vi "信号发生器（配置文件1）.vi"() -> ()   [LabVIEW 2020]
uses:
  <vilib>/Utility/xml.llb/Read From XML File(string).vi
  <vilib>/Utility/config.llb/Read Key (I32).vi
  <vilib>/Utility/config.llb/Read Key (Double).vi
  <vilib>/Utility/config.llb/Read Key (Boolean).vi
  <vilib>/Utility/xml.llb/Write to XML File(string).vi
  <vilib>/Utility/config.llb/Write Key (U32).vi
  <vilib>/Utility/config.llb/Write Key (Double).vi
  <vilib>/Utility/config.llb/Write Key (Boolean).vi
  <vilib>/measure/NI_MABase.lvlib
  <vilib>/Utility/config.llb/NI_LVConfig.lvlib
panel:
  out "Hall Channel 1":waveform(dbl)(graph)
  out "车型数组":string[](array[string])
  in  "STOP":bool
  in  "AO3 Channel":u32(ring)=4 items=["Hall Channel 1", "Hall Channel 2", "ME Channel 1", "ME Channel 2", "ME Channel 3", "ME Channel 4"]
  in  "AO2 Channel":u32(ring)=3 items=["ME Channel 1", "ME Channel 2", "ME Channel 1", "ME Channel 2", "ME Channel 3", "ME Channel 4"]
  in  "AO1 Channel":u32(ring)=2 items=["Hall Channel 1", "Hall Channel 2", "ME Channel 1", "ME Channel 2", "ME Channel 3", "ME Channel 4"]
  in  "AO0 Channel":u32(ring) items=["Hall Channel 1", "Hall Channel 2", "ME Channel 1", "ME Channel 2", "ME Channel 3", "ME Channel 4"]
  out "转速表":dbl(knob) scale=0.0..3000.0
  in  "Speed FM":dbl(knob)=583.5936811226446 caption="转速调频" scale=50.0..1000.0
  in  "Brand":u32(ring)=2 items=["卡特", "凯斯", "日立", "神钢", "沃尔沃", "现代", "小松", "住友", "三一"]
  in  "Vehicle models":u32(ring) items=["五十铃6HK1", "五十铃6WG1", "五十铃新版4HK1"]
  out "ME Channel 4":waveform(dbl)(graph)
  out "ME Channel 3":dynamicdata(graph)
  out "ME Channel 2":waveform(dbl)(graph)
  out "ME Channel 1":dynamicdata(graph)
  out "Hall Channel 2":waveform(dbl)(graph)
  out "数组大小":i32
  out "品牌":string
  out "品牌数组":string[](array[string])
  in  "error":errorcluster caption="错误输入（无错误）"
  in  "字符串数组类型":string[](array[string])
  out "数值合法":bool
  out "凸轮轴参数":T1
  out "0凸轮轴信号类型":u32
  out "0凸轮轴电压幅值":dbl format="%#.1f"
  out "0信号个数":dbl=7.0 caption="信号个数" format="%#.1f"
  out "0凸轮轴个数":dbl=1.0 caption="凸轮轴个数" format="%#.1f"
  out "0凸轮轴是否取反":bool
  out "0凸轮轴周期":dbl=3.0 caption="凸轮轴周期" format="%#.1f"
  out "0起始偏移":dbl=3.0 caption="凸轮轴周期" format="%#.1f"
  out "0插齿间隔":dbl=3.0 caption="凸轮轴周期" format="%#.1f"
  out "0间隔齿数":dbl=3.0 caption="凸轮轴周期" format="%#.1f"
  out "曲轴参数":T2
  out "0曲轴轴信号类型":u32
  out "0曲轴电压幅值":dbl format="%#.1f"
  out "0总齿数":dbl=7.0 caption="信号个数" format="%#.1f"
  out "0曲轴个数":dbl=1.0 caption="凸轮轴个数" format="%#.1f"
  out "0曲轴是否取反":bool
  out "0缺齿数":dbl=3.0 caption="凸轮轴周期" format="%#.1f"
  out "0曲轴圈数":dbl=3.0 caption="凸轮轴周期" format="%#.1f"
  out "0缺齿偏移":dbl=3.0 caption="凸轮轴周期" format="%#.1f"
  out "品牌车型数组":string[](array[string])
  out "凸轮轴信号类型":u16(ring) items=["磁电式", "霍尔式", "无曲轴"]
  out "曲轴圈数信号":dynamicdata(graph)
  out "1缺齿偏移":dbl=4.0
  out "缺齿偏移":dbl=8.2 format="%_2f"
  out "长平组信号正弦":dynamicdata(graph)
  out "间隔长平+正弦信号":dynamicdata(graph)
  out "曲轴组合波形":waveform(dbl)(graph)
  out "1曲轴圈数":dbl=4.0
  out "曲轴圈数":dbl=8.2
  out "长平组信号":dynamicdata(graph)
  out "间隔长平+凸信号":dynamicdata(graph)
  out "间隔齿数":dbl=3.0
  out "1间隔齿数":dbl=3.0 caption="凸轮轴周期"
  out "1插齿间隔":dbl=3.0 caption="凸轮轴周期"
  out "1起始偏移":dbl=3.0 caption="凸轮轴周期"
  out "插齿间隔":dbl=8.2
  out "起始偏移":dbl=8.2
  out "车型数组大小":i32
  in  "error":errorcluster caption="错误输入（无错误）"
  in  "字符串数组类型":string[](array[string])
  out "凸轮轴周期·":dbl=8.2 caption="凸轮轴周期"
  out "凸轮轴个数":dbl=8.2
  out "曲轴个数":dbl=8.2
  out "信号个数":dbl=8.2
  out "凸轮轴是否取反":bool
  out "凸轮轴电压幅值":dbl=8.2 format="%0.2p"
  out "曲轴是否取反":bool
  out "曲轴信号类型":u16(ring) items=["磁电式", "霍尔式", "无曲轴"]
  out "缺齿数":dbl=4.0
  out "总齿数":dbl=60.0
  out "曲轴电压幅值":dbl=8.2 format="%0.2p"
  out "1凸轮轴周期·":dbl=3.0 caption="凸轮轴周期"
  out "1凸轮轴是否取反":bool
  out "1凸轮轴个数":dbl=1.0 caption="凸轮轴个数"
  out "1信号个数":dbl=7.0 caption="信号个数"
  out "1凸轮轴电压幅值":dbl=5.0 caption="凸轮轴电压幅值" format="%0.2p"
  out "1凸轮轴信号类型":u16(ring)=1 items=["磁电式", "霍尔式", "无凸轮轴"]
  out "1缺齿数":dbl=4.0
  out "1总齿数":dbl=60.0
  out "1曲轴个数":dbl=2.0 caption="曲轴个数"
  out "1曲轴是否取反":bool
  out "1曲轴电压幅值":dbl=18.0 caption="曲轴电压幅值" format="%0.2p"
  out "1曲轴信号类型":u16(ring) items=["磁电式", "霍尔式", "无曲轴"]
  out "1波形图":waveform(dbl)(graph)
  out "起始偏移（方波）":dbl
  out "起始偏移（正弦）":dbl=0.5
  out "中短平+2正弦":dynamicdata(graph)
  out "长平+1正弦":dynamicdata(graph)
  out "长水平线数量（正弦）":dbl
  out "一个正弦波形图":waveform(dbl)(graph)
  out "起始水平线个数（正弦）":dbl
  out "起始平+1正弦":dynamicdata(graph)
  out "6波形图":waveform(dbl)(graph)
  out "5波形图":waveform(dbl)(graph)
  out "起始水平线个数（方波）":dbl
  out "长平+1凸":dynamicdata(graph)
  out "长水平线数量（方波）":dbl
  out "曲轴":dynamicdata(graph)
  out "曲轴方波缺齿波形图":dynamicdata(graph)
  out "曲轴方波偏移量":dbl=8.2 format="%0.2p"
  out "曲轴方波波形图":waveform(dbl)(graph)
  out "中、短平+2凸":dynamicdata(graph)
  out "起始平+1凸":dynamicdata(graph)
  out "一个凸起波形图":dynamicdata(graph)
  out "曲轴正弦偏移量":dbl caption="偏移量" format="%0.2p"
  out "曲轴正弦波形图":waveform(dbl)(graph)
  out "完\n整\n缺\n齿\n波":waveform(dbl)(graph)
  out "未\n翻\n转\n半\n缺\n齿":dynamicdata(graph)
  out "圆\n弧\n+\n水\n平":dynamicdata(graph)
  out "半\n缺\n齿\n水\n平\n线":waveform(dbl)(graph)
  out "圆\n弧":waveform(dbl)(graph)
  out "t0":timestamp
  out "x轴取点间隔":dbl
  out "循环次数":i32
  out "圆弧点数":dbl=33.0 format="%0.2p"
  out "dt":dbl
  out "圆半径":dbl=2.48 format="%0.2p"
  out "部分\n正弦\n波形图":waveform(dbl)(graph)
  in  "波形发生率Fs":dbl=50000.0
types:
  T1 = cluster{"0凸轮轴信号类型":u32, "0凸轮轴电压幅值":dbl, "0信号个数":dbl, "0凸轮轴个数":dbl, "0凸轮轴是否取反":bool, "0凸轮轴周期":dbl, "0起始偏移":dbl, "0插齿间隔":dbl, "0间隔齿数":dbl}
  T2 = cluster{"0曲轴轴信号类型":u32, "0曲轴电压幅值":dbl, "0总齿数":dbl, "0曲轴个数":dbl, "0曲轴是否取反":bool, "0却齿数":dbl, "0曲轴圈数":dbl, "0缺齿偏移":dbl}
  T3 = typedef "NI_LVConfig.lvlib/Config Data RefNum.ctl" = refnum<k1>
  T4 = cluster{"0曲轴轴信号类型":u32, "0曲轴电压幅值":dbl, "0总齿数":dbl, "0曲轴个数":dbl, "0曲轴是否取反":bool, "0缺齿数":dbl, "0曲轴圈数":dbl, "0缺齿偏移":dbl}
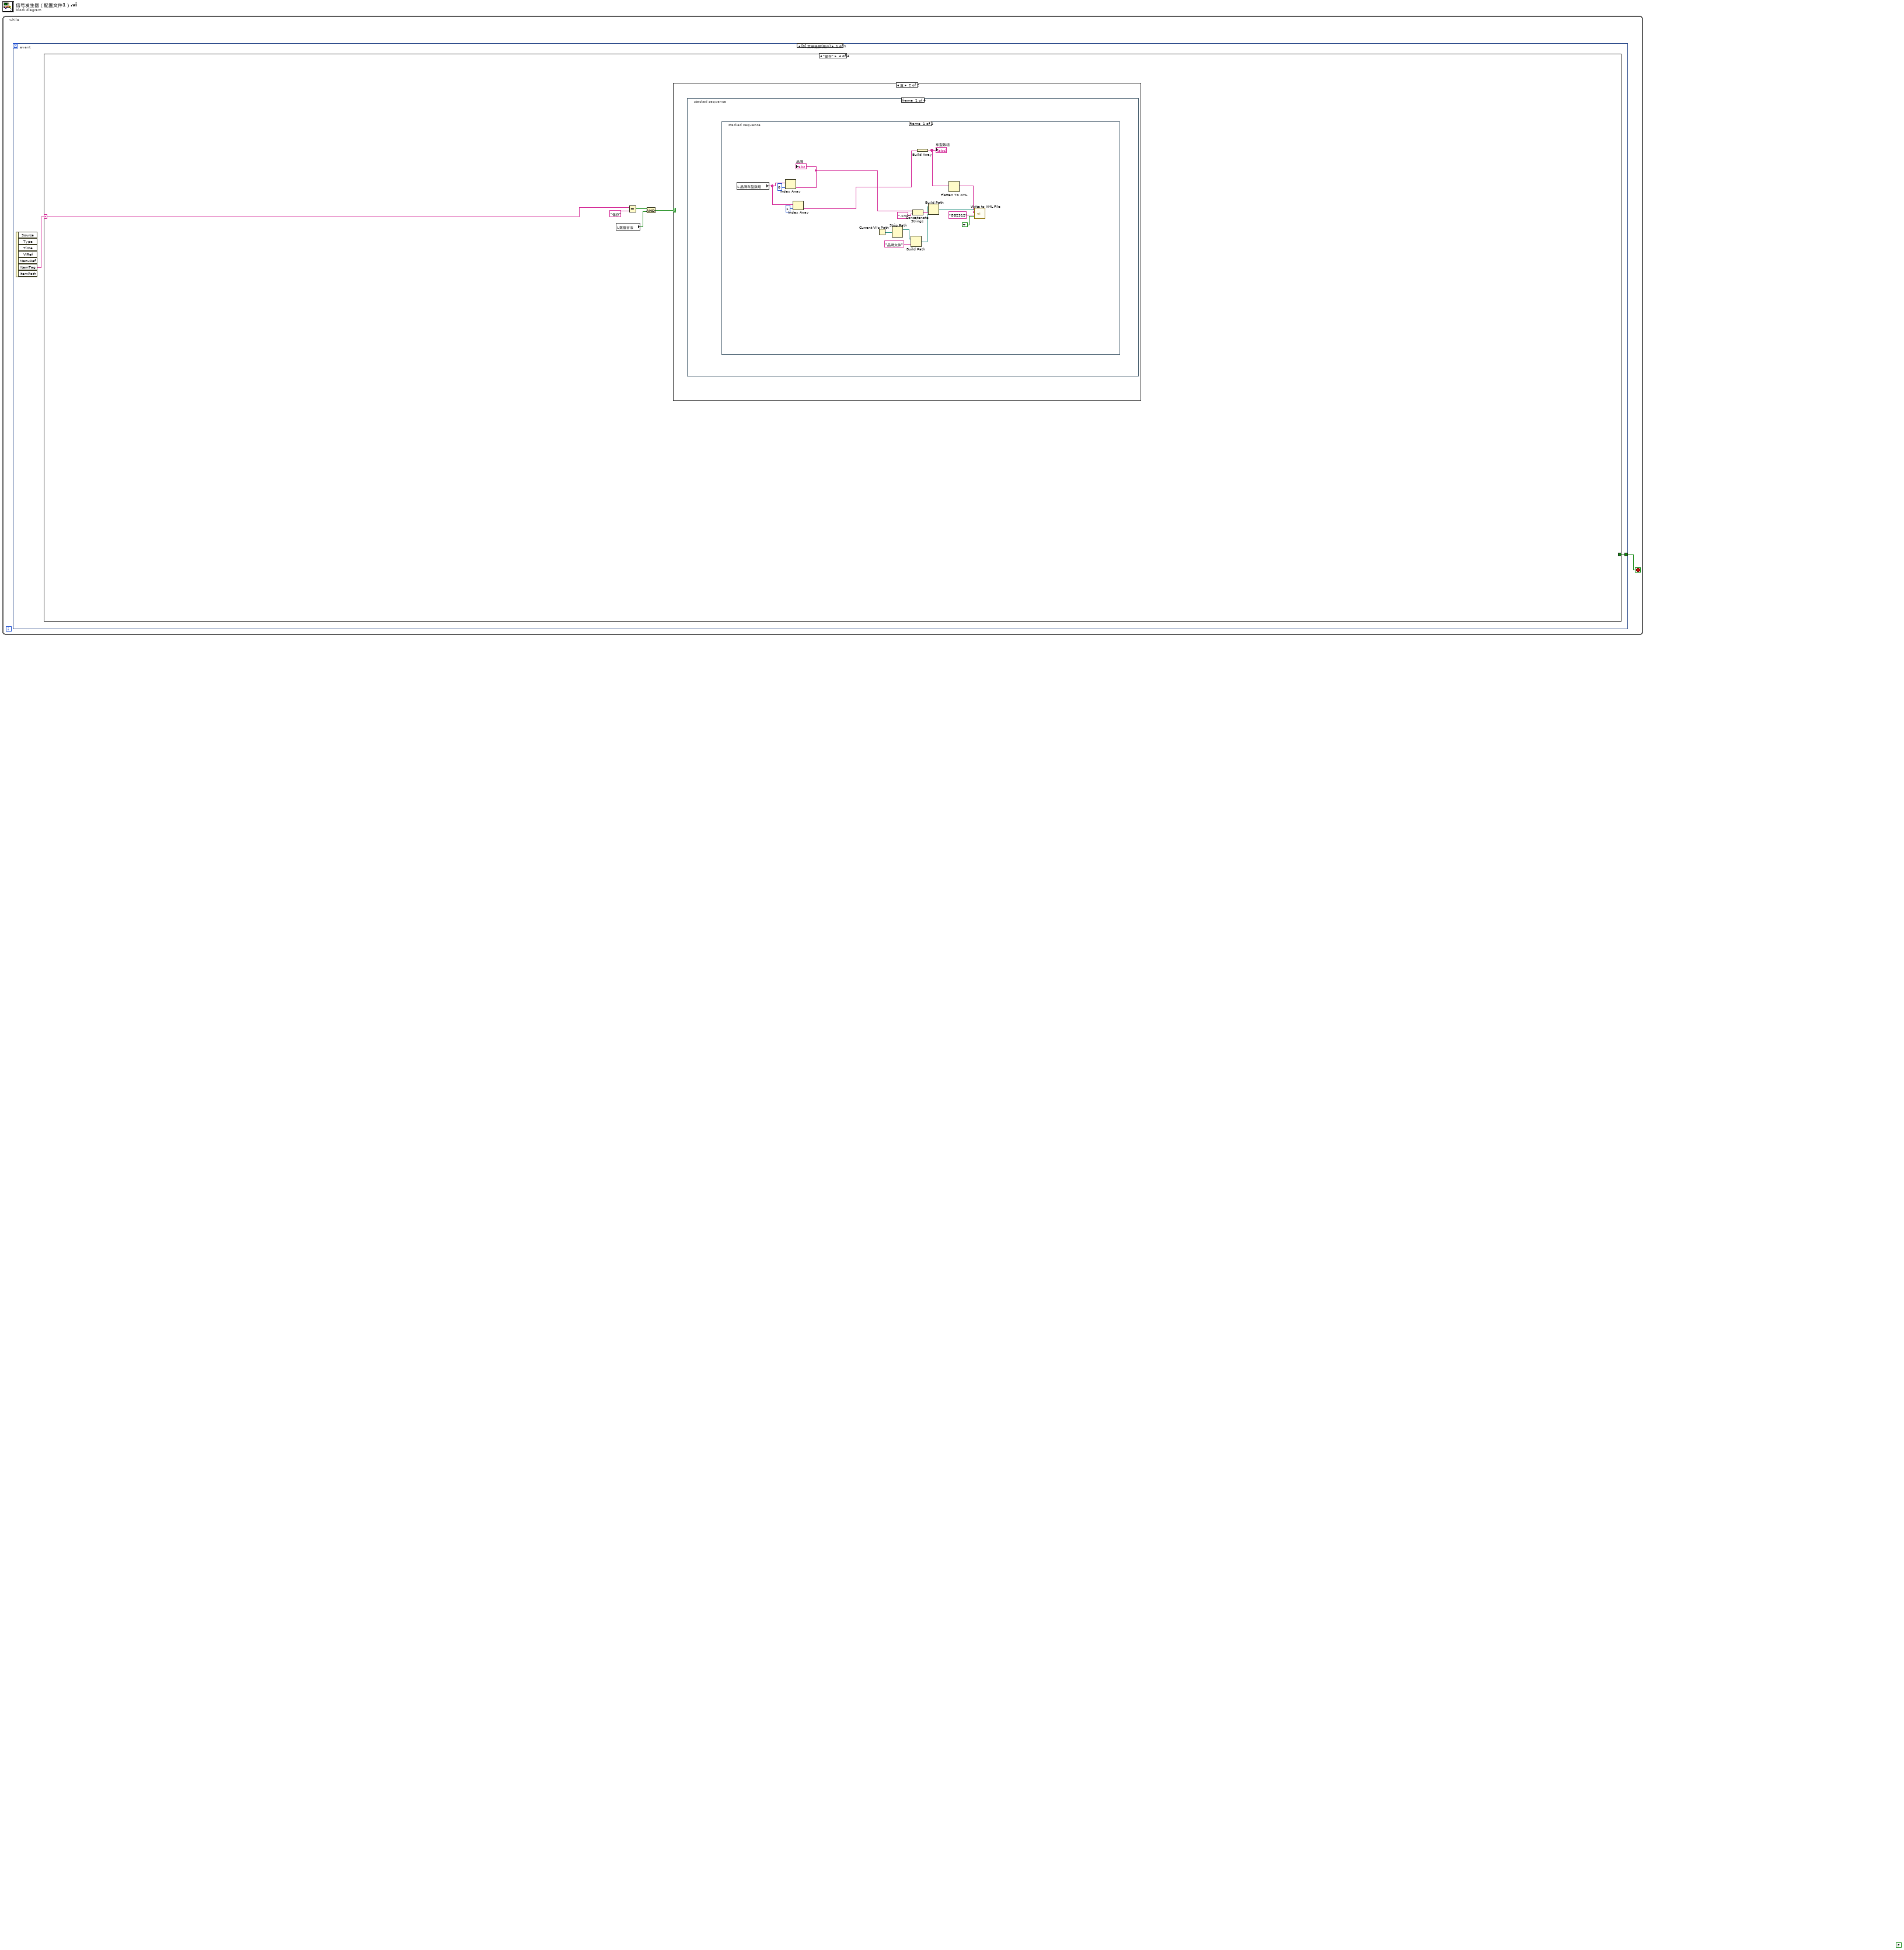
[diagram p0: block diagram]
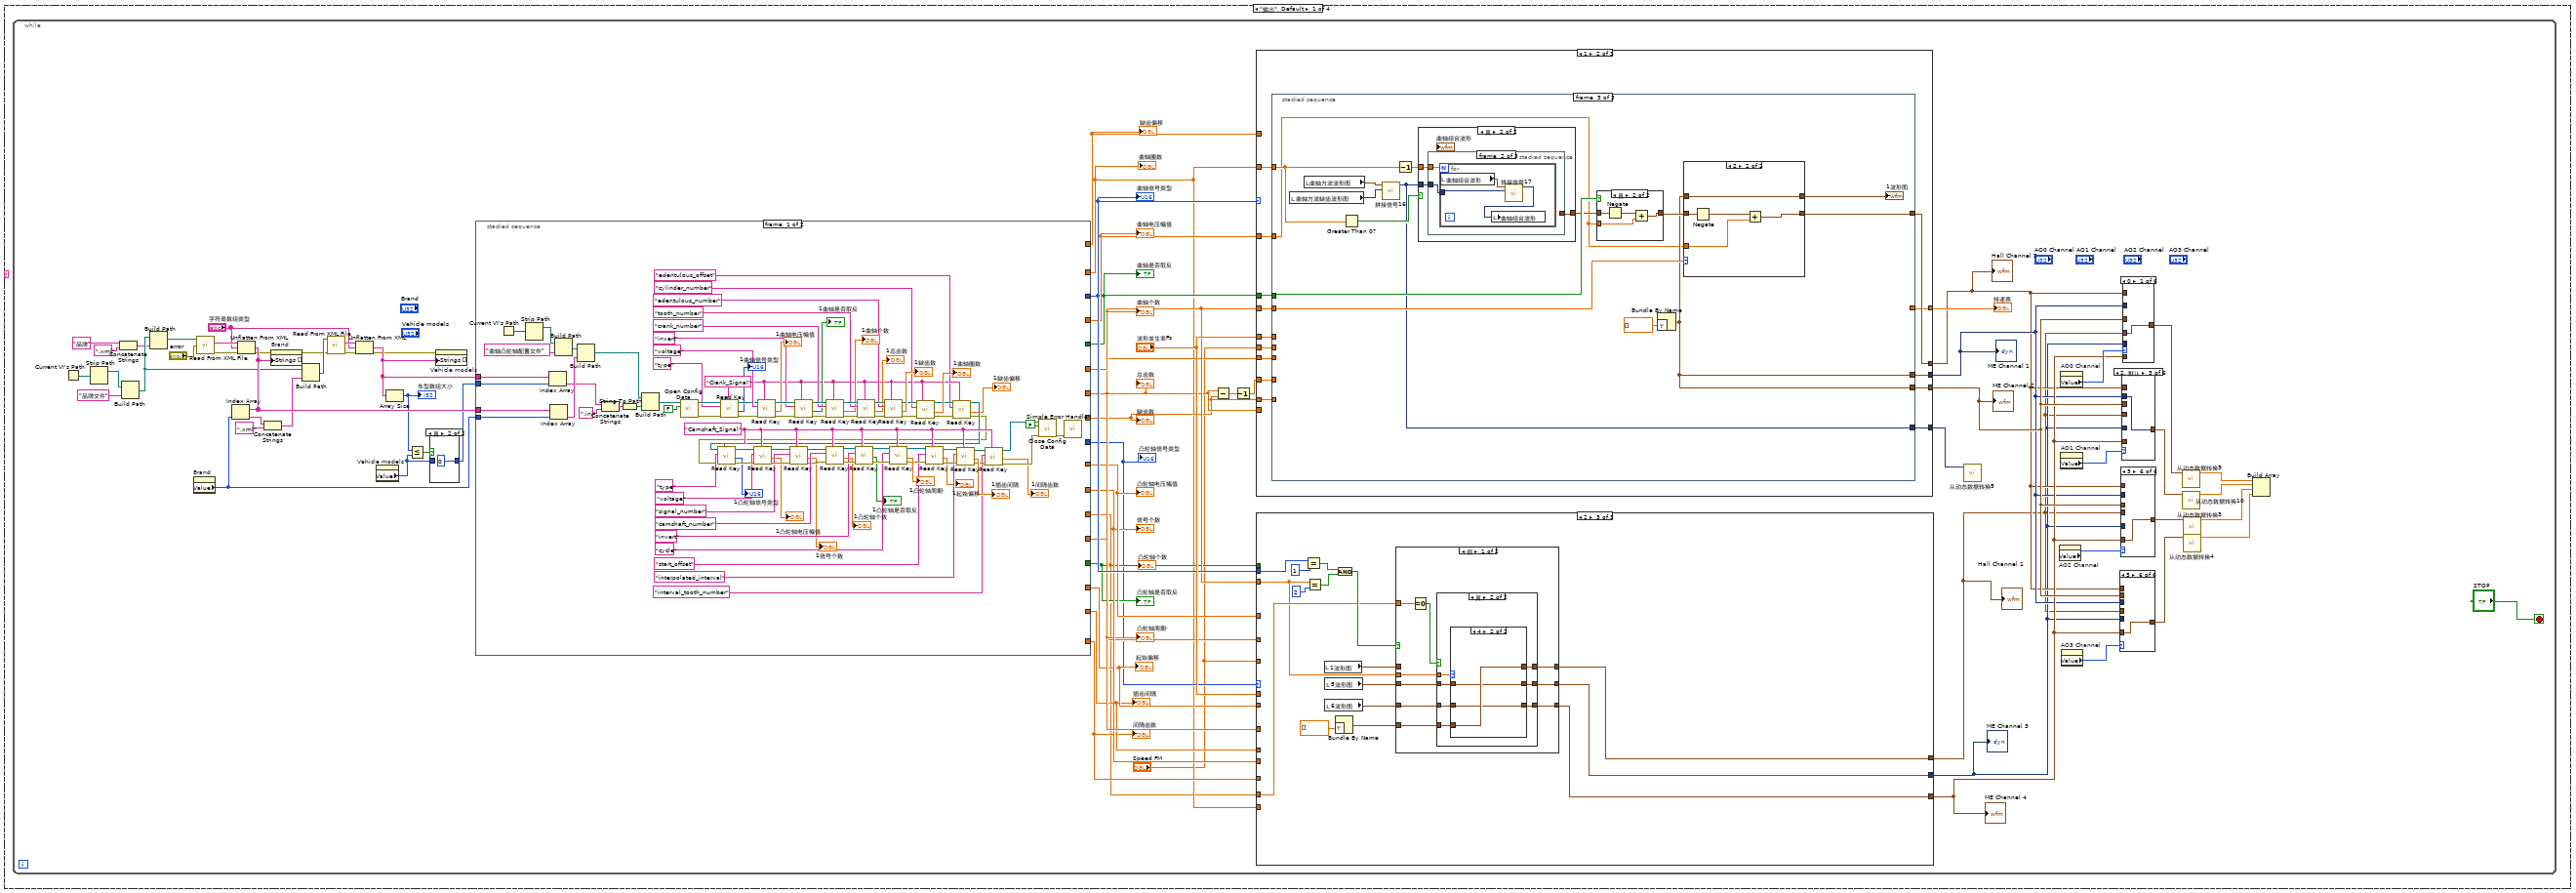
[diagram p2: hidden frame]
diagram:
  (unwired) FALSE
  n1 = while {
    stop <- w1 stop-if-true
    n2 = event shown="[0] 菜单选择(用户)" {
      selector: _ -> [_]
      dyn-events: _ -> [_]
      timeout: _ -> [_]
      tunnel: [w3] -> w1
      event Menu Selection (User) {
        n3 = event-data() -> ("ItemTag"=w2:string)  [unwired: 1 in, 6 out]
        n4 = case shown="\"保存\"" w2 {
          selector: w2 -> [_ _ _ w1190]
          tunnel: [_ TRUE _ _] -> w3
          frame "输出", Default {
            n5 = while {
              stop <- "STOP" stop-if-true
              n6 = Current VI's Path() -> (path=w53:path)
              n7 = Strip Path(path=w53) -> (stripped path=w52:path)  [unwired: 1 out]
              n8 = Concatenate Strings("品牌" ("字符串"), ".xml") -> (w43:string)
              n9 = Build Path(base path=w52, name or relative path="品牌文件" ("名称或相对路径")) -> (appended path=w44:path)
              n10 = Build Path(base path=w44, name or relative path=w43) -> (appended path=w42:path)
              n11 = property on="Brand" class="Ring (严格)"() -> ("Value"=w59:u32)  [unwired: 2 in, 2 out]
              n12 = call-poly <vilib>:"Read From XML File.vi"("error in (no error)"="error", "XML File Path"=w42) -> ("error out"=w56:errorcluster, "XML Elements"=w55:string)  [unwired: 7 in, 1 out]
              n13 = Unflatten From XML(xml string=w55, type="字符串数组类型", error in (no error)=w56) -> (value=w60:string[], error out=w48:errorcluster)
              n14 = Index Array(array=w60, index=w59) -> (element=w54:string)
              n15 = Concatenate Strings(w54, ".xml") -> (w51:string)
              n16 = property on="Brand" class="Ring (严格)"(error in=w48, "Strings []"=w60) -> (error out=w13:errorcluster)  [unwired: 1 in, 1 out]
              n17 = Build Path(base path=w44, name or relative path=w51) -> (appended path=w37:path)
              n18 = call-poly <vilib>:"Read From XML File.vi"("error in (no error)"=w13, "XML File Path"=w37) -> ("error out"=w41:errorcluster, "XML Elements"=w40:string)  [unwired: 7 in, 1 out]
              n19 = Unflatten From XML(xml string=w40, type="字符串数组类型", error in (no error)=w41) -> (value=w58:string[], error out=w39:errorcluster)
              n20 = property on="Vehicle models" class="Ring (严格)"() -> ("Value"=w35:u32)  [unwired: 2 in, 2 out]
              n21 = Array Size(array=w58) -> (size(s)=w34:i32)
              "车型数组大小" <- w34
              n22 = Less Or Equal?(x=w34, y=w35) -> (x <= y?=w36:bool)
              n23 = case shown="真" w36 {
                tunnel: w35 -> [w98 _]
                tunnel: [w98 0] -> w57
                frame False {
                }
                frame True {
                }
              }
              n24 = property on="Vehicle models" class="Ring (严格)"(error in=w39, "Strings []"=w58) -> ()  [unwired: 1 in, 2 out]
              n25 = stacked-sequence {
                tunnel: [_ w206] -> w70
                tunnel: [_ w205] -> w69
                tunnel: [_ w204] -> w68
                tunnel: [_ w203] -> w67
                tunnel: [_ w202] -> w66
                tunnel: [_ w201] -> w65
                tunnel: [_ w200] -> w22
                tunnel: [_ w199] -> w64
                tunnel: [_ w198] -> w63
                tunnel: [_ w197] -> w10
                tunnel: [_ w196] -> w62
                tunnel: [_ w195] -> w61
                tunnel: w60 -> [w134 _]
                tunnel: w58 -> [w131 _]
                tunnel: w59 -> [w127 _]
                tunnel: w57 -> [w126 _]
                tunnel: [_ w194] -> w33
                tunnel: [_ w193] -> w32
                tunnel: [_ w192] -> w31
                tunnel: [_ w191] -> w11
                tunnel: [_ w190] -> w30
                frame #0 {
                  w113 = "Camshaft_Signal" ("section")
                  w103 = "Crank_Signal" ("section")
                  n26 = Current VI's Path() -> (path=w140:path)
                  n27 = Strip Path(path=w140) -> (stripped path=w139:path)  [unwired: 1 out]
                  n28 = Index Array(array=w131, index=w126) -> (element=w130:string)
                  n29 = Index Array(array=w134, index=w127) -> (element=w133:string)
                  n30 = Build Path(base path=w139, name or relative path="曲轴凸轮轴配置文件" ("名称或相对路径")) -> (appended path=w135:path)
                  n31 = Build Path(base path=w135, name or relative path=w133) -> (appended path=w136:path)
                  n32 = Concatenate Strings(w130, ".ini" ("字符串")) -> (w128:string)
                  n33 = String To Path(string=w128) -> (path=w129:path)
                  n34 = Build Path(base path=w136, name or relative path=w129) -> (appended path=w137:path)
                  n35 = call <vilib>:"Open Config Data.vi"("create file if necessary (T)"=FALSE ("create file if necessary? (T)"), "configuration file path"=w137) -> ("error out"=w169:errorcluster, "refnum"=w167:T3)  [unwired: 7 in, 1 out]
                  n36 = call-poly <vilib>:"Read Key.vi"("section"=w103, "error in (no error)"=w169, "key"="type", "refnum"=w167) -> ("error out"=w170:errorcluster, "value"=→"1曲轴信号类型":i32, "refnum out"=w168:T3)  [unwired: 1 in, 4 out]
                  n37 = call-poly <vilib>:"Read Key.vi"("section"=w103, "error in (no error)"=w170, "key"="voltage" ("键2"), "refnum"=w168) -> ("error out"=w165:errorcluster, "value"=→"1曲轴电压幅值":dbl, "refnum out"=w164:T3)  [unwired: 1 in, 4 out]
                  n38 = call-poly <vilib>:"Read Key.vi"("section"=w103, "error in (no error)"=w165, "key"="invert" ("键3"), "refnum"=w164) -> ("error out"=w162:errorcluster, "value"=→"1曲轴是否取反":bool, "refnum out"=w161:T3)  [unwired: 1 in, 4 out]
                  n39 = call-poly <vilib>:"Read Key.vi"("section"=w103, "error in (no error)"=w162, "key"="crank_number" ("键3"), "refnum"=w161) -> ("error out"=w159:errorcluster, "value"=→"1曲轴个数":dbl, "refnum out"=w158:T3)  [unwired: 1 in, 4 out]
                  n40 = call-poly <vilib>:"Read Key.vi"("section"=w103, "error in (no error)"=w159, "key"="tooth_number" ("键3"), "refnum"=w158) -> ("error out"=w156:errorcluster, "value"=→"1总齿数":dbl, "refnum out"=w157:T3)  [unwired: 1 in, 4 out]
                  n41 = call-poly <vilib>:"Read Key.vi"("section"=w103, "error in (no error)"=w156, "key"="edentulous_number" ("键3"), "refnum"=w157) -> ("error out"=w109:errorcluster, "value"=→"1缺齿数":dbl, "refnum out"=w108:T3)  [unwired: 1 in, 4 out]
                  n42 = call-poly <vilib>:"Read Key.vi"("section"=w103, "error in (no error)"=w109, "key"="cylinder_number" ("键3"), "refnum"=w108) -> ("error out"=w102:errorcluster, "value"=→"1曲轴圈数":dbl, "refnum out"=w105:T3)  [unwired: 1 in, 4 out]
                  n43 = call-poly <vilib>:"Read Key.vi"("section"=w103, "error in (no error)"=w102, "key"="edentulous_offset" ("键2"), "refnum"=w105) -> ("error out"=w101:errorcluster, "value"=→"1缺齿偏移":dbl, "refnum out"=w106:T3)  [unwired: 1 in, 4 out]
                  n44 = call-poly <vilib>:"Read Key.vi"("section"=w113, "error in (no error)"=w101, "key"="type" ("键3"), "refnum"=w106) -> ("error out"=w189:errorcluster, "value"=→"1凸轮轴信号类型":i32, "refnum out"=w188:T3)  [unwired: 2 in, 3 out]
                  n45 = call-poly <vilib>:"Read Key.vi"("section"=w113, "error in (no error)"=w189, "key"="voltage" ("键3"), "refnum"=w188) -> ("error out"=w182:errorcluster, "value"=→"1凸轮轴电压幅值":dbl, "refnum out"=w180:T3)  [unwired: 2 in, 3 out]
                  n46 = call-poly <vilib>:"Read Key.vi"("section"=w113, "error in (no error)"=w182, "key"="signal_number" ("键3"), "refnum"=w180) -> ("error out"=w145:errorcluster, "value"=→"1信号个数":dbl, "refnum out"=w179:T3)  [unwired: 2 in, 3 out]
                  n47 = call-poly <vilib>:"Read Key.vi"("section"=w113, "error in (no error)"=w145, "key"="camshaft_number" ("键3"), "refnum"=w179) -> ("error out"=w181:errorcluster, "value"=→"1凸轮轴个数":dbl, "refnum out"=w178:T3)  [unwired: 2 in, 3 out]
                  n48 = call-poly <vilib>:"Read Key.vi"("section"=w113, "error in (no error)"=w181, "key"="invert" ("键2"), "refnum"=w178) -> ("error out"=w183:errorcluster, "value"=→"1凸轮轴是否取反":bool, "refnum out"=w177:T3)  [unwired: 2 in, 3 out]
                  n49 = call-poly <vilib>:"Read Key.vi"("section"=w113, "error in (no error)"=w183, "key"="cycle", "refnum"=w177) -> ("error out"=w122:errorcluster, "value"=→"1凸轮轴周期·":dbl, "refnum out"=w125:T3)  [unwired: 2 in, 3 out]
                  n50 = call-poly <vilib>:"Read Key.vi"("section"=w113, "error in (no error)"=w122, "key"="start_offset" ("键2"), "refnum"=w125) -> ("error out"=w123:errorcluster, "value"=→"1起始偏移":dbl, "refnum out"=w124:T3)  [unwired: 2 in, 3 out]
                  n51 = call-poly <vilib>:"Read Key.vi"("section"=w113, "error in (no error)"=w123, "key"="interpolated_interval", "refnum"=w124) -> ("error out"=w116:errorcluster, "value"=→"1插齿间隔":dbl, "refnum out"=w117:T3)  [unwired: 2 in, 3 out]
                  n52 = call-poly <vilib>:"Read Key.vi"("section"=w113, "error in (no error)"=w116, "key"="interval_tooth_number", "refnum"=w117) -> ("error out"=w115:errorcluster, "value"=→"1间隔齿数":dbl, "refnum out"=w114:T3)  [unwired: 2 in, 3 out]
                  n53 = call <vilib>:"Close Config Data.vi"("error in (no error)"=w115, "write file if changed (T)"=FALSE ("write configuration file? (T)"), "refnum"=w114) -> ("error out"=w184:errorcluster)  [unwired: 8 out]
                  n54 = call <vilib>:"Simple Error Handler.vi"("error in (no error)"=w184) -> ()  [unwired: 1 in, 8 out]
                }
                frame #1 {
                  n55 = local read "1缺齿偏移"() -> (w190:dbl)
                  n56 = local read "1曲轴圈数"() -> (w191:dbl)
                  n57 = local read "1曲轴信号类型"() -> (w206:u16)
                  n58 = local read "1曲轴电压幅值"() -> (w205:dbl)
                  n59 = local read "1曲轴是否取反"() -> (w204:bool)
                  n60 = local read "1曲轴个数"() -> (w203:dbl)
                  n61 = local read "1总齿数"() -> (w202:dbl)
                  n62 = local read "1缺齿数"() -> (w201:dbl)
                  n63 = local read "1凸轮轴信号类型"() -> (w200:u16)
                  n64 = local read "1凸轮轴电压幅值"() -> (w199:dbl)
                  n65 = local read "1信号个数"() -> (w198:dbl)
                  n66 = local read "1凸轮轴个数"() -> (w197:dbl)
                  n67 = local read "1凸轮轴周期·"() -> (w195:dbl)
                  n68 = local read "1凸轮轴是否取反"() -> (w196:bool)
                  n69 = local read "1起始偏移"() -> (w194:dbl)
                  n70 = local read "1插齿间隔"() -> (w193:dbl)
                  n71 = local read "1间隔齿数"() -> (w192:dbl)
                }
              }
              "总齿数" <- w66
              "缺齿数" <- w65
              "曲轴信号类型" <- w70
              "曲轴电压幅值" <- w69
              "曲轴是否取反" <- w68
              "凸轮轴电压幅值" <- w64
              "凸轮轴是否取反" <- w62
              "信号个数" <- w63
              "曲轴个数" <- w67
              "凸轮轴个数" <- w10
              "凸轮轴周期·" <- w61
              "起始偏移" <- w33
              "插齿间隔" <- w32
              "间隔齿数" <- w31
              "曲轴圈数" <- w11
              "缺齿偏移" <- w30
              "凸轮轴信号类型" <- w22
              n72 = Subtract(x=w66, y=w65) -> (x-y=w73:dbl)
              n73 = Decrement(x=w73) -> (x-1=w72:dbl)
              n74 = case shown="2" w22 {
                tunnel: "Speed FM" -> [w220 w398 _]
                tunnel: "波形发生率Fs" -> [w219 w397 _]
                tunnel: w66 -> [w218 w396 _]
                tunnel: w64 -> [w221 w395 _]
                tunnel: [w212 w394 w644] -> w4
                tunnel: w63 -> [w217 w393 _]
                tunnel: [w213 w392 w641] -> w20
                tunnel: [w214 w391 w640] -> w6
                tunnel: w61 -> [w216 w387 _]
                tunnel: w10 -> [w215 w390 w639]
                tunnel: w70 -> [_ _ w651]
                tunnel: w67 -> [_ _ w636]
                tunnel: w62 -> [w211 w389 _]
                tunnel: w33 -> [w210 w384 _]
                tunnel: w32 -> [w209 w385 _]
                tunnel: w31 -> [w207 w383 _]
                tunnel: w11 -> [w208 _ _]
                frame 0, Default {
                  n75 = stacked-sequence {
                    tunnel: w221 -> [w249 _ _ w327]
                    tunnel: w220 -> [w231 w260 w284 w339]
                    tunnel: w219 -> [w238 w259 w283 w340]
                    tunnel: w218 -> [w246 _ _ _]
                    tunnel: w217 -> [w247 _ _ w312]
                    tunnel: w216 -> [w229 _ w276 _]
                    tunnel: w215 -> [_ _ _ w331]
                    tunnel: [_ _ _ w330] -> w214
                    tunnel: [_ _ _ w328] -> w213
                    tunnel: [_ _ _ w325] -> w212
                    tunnel: w211 -> [_ _ _ w321]
                    tunnel: w210 -> [w224 w255 _ _]
                    tunnel: w209 -> [_ _ w273 _]
                    tunnel: w208 -> [w222 _ _ _]
                    tunnel: w207 -> [_ _ _ w311]
                    frame #0 {
                      n76 = Divide(x=w231, y=w229) -> (x/y=w230:dbl)
                      n77 = Decrement(x=w247) -> (x-1=w223:dbl)
                      n78 = Divide(x=w249, y=2.0) -> (x/y=w237:dbl)
                      n79 = Divide(x=w238, y=w230) -> (x/y=w248:dbl)
                      n80 = Multiply(x=w246, y=w222) -> (x*y=w228:dbl)
                      n81 = Multiply(x=w229, y=w223) -> (x*y=w227:dbl)
                      n82 = Subtract(x=w228, y=w227) -> (x-y=w226:dbl)
                      n83 = Bundle By Name(cluster=cluster{"Fs":dbl, "#s":dbl} {"Fs"=1000.0, "#s"=1000.0} ("sampling info"), "Fs"=w238, "#s"=w248) -> (w253:cluster{"Fs":dbl, "#s":dbl})
                      n84 = Divide(x=w226, y=w223) -> (x/y=w225:dbl)
                      n85 = Subtract(x=w225, y=w224) -> (x-y=w239:dbl)
                      "起始水平线个数（正弦）" <- w239
                      n86 = call <vilib>:"Sine Waveform.vi"("offset"=0.0, "sampling info"=w253, "reset signal"=TRUE, "amplitude"=w237, "frequency"=w230) -> ("signal out"=w232:waveform(dbl))  [unwired: 5 in, 1 out]
                      "一个正弦波形图" <- w232
                      n87 = Divide(x=w238, y=w231) -> (x/y=w243:dbl)
                      n88 = Multiply(x=w243, y=w239) -> (x*y=w242:dbl)
                      n89 = Bundle By Name(cluster=cluster{"Fs":dbl, "#s":dbl} {"Fs"=1000.0, "#s"=1000.0} ("sampling info"), "Fs"=w238, "#s"=w242) -> (w244:cluster{"Fs":dbl, "#s":dbl})
                      n90 = call <vilib>:"Square Waveform.vi"("duty cycle (%)"=0.0, "offset"=0.0, "sampling info"=w244, "reset signal"=TRUE, "amplitude"=0.0, "frequency"=w231) -> ("signal out"=w235:waveform(dbl))  [unwired: 4 in, 1 out]
                      n91 = call "拼接信号25"("Input Signal B"=w232, "Input Signal A"=w235) -> ("Appended Signals"=→"起始平+1正弦":dynamicdata)  [unwired: 8 in, 1 out]
                      "起始偏移（正弦）" <- w224
                    }
                    frame #1 {
                      n92 = local read "起始水平线个数（正弦）"() -> (w270:dbl)
                      n93 = Divide(x=w259, y=w260) -> (x/y=w267:dbl)
                      n94 = Add(x=w270, y=w255) -> (x+y=w261:dbl)
                      "长水平线数量（正弦）" <- w261
                      n95 = Multiply(x=w267, y=w261) -> (x*y=w266:dbl)
                      n96 = Bundle By Name(cluster=cluster{"Fs":dbl, "#s":dbl} {"Fs"=1000.0, "#s"=1000.0} ("sampling info"), "Fs"=w259, "#s"=w266) -> (w268:cluster{"Fs":dbl, "#s":dbl})
                      n97 = call <vilib>:"Square Waveform.vi"("duty cycle (%)"=0.0, "offset"=0.0, "sampling info"=w268, "reset signal"=TRUE, "amplitude"=0.0, "frequency"=w260) -> ("signal out"=w258:waveform(dbl))  [unwired: 4 in, 1 out]
                      n98 = local read "一个正弦波形图"() -> (w257:waveform(dbl))
                      n99 = call "拼接信号26"("Input Signal B"=w257, "Input Signal A"=w258) -> ("Appended Signals"=→"长平+1正弦":dynamicdata)  [unwired: 8 in, 1 out]
                    }
                    frame #2 {
                      n100 = local read "长水平线数量（正弦）"() -> (w282:dbl)
                      n101 = local read "一个正弦波形图"() -> (w272:waveform(dbl))
                      n102 = Equal To 0?(x=w273) -> (x = 0?=w274:bool)
                      n103 = Subtract(x=w282, y=w276) -> (x-y=w275:dbl)
                      n104 = case shown="假" w274 {
                        tunnel: w284 -> [_ w299]
                        tunnel: w283 -> [_ w298]
                        tunnel: w273 -> [_ w297]
                        tunnel: w272 -> [w293 w296]
                        tunnel: [w293 w294] -> w271
                        frame True {
                        }
                        frame False {
                          n105 = Divide(x=w298, y=w299) -> (x/y=w305:dbl)
                          n106 = Multiply(x=w305, y=w297) -> (x*y=w304:dbl)
                          n107 = Bundle By Name(cluster=cluster{"Fs":dbl, "#s":dbl} {"Fs"=1000.0, "#s"=1000.0} ("sampling info"), "Fs"=w298, "#s"=w304) -> (w306:cluster{"Fs":dbl, "#s":dbl})
                          n108 = call <vilib>:"Square Waveform.vi"("duty cycle (%)"=0.0, "offset"=0.0, "sampling info"=w306, "reset signal"=TRUE, "amplitude"=0.0, "frequency"=w299) -> ("signal out"=w295:waveform(dbl))  [unwired: 4 in, 1 out]
                          n109 = call "拼接信号28"("Input Signal B"=w296, "Input Signal A"=w295) -> ("Appended Signals"=w294:dynamicdata)  [unwired: 8 in, 1 out]
                        }
                      }
                      n110 = Divide(x=w283, y=w284) -> (x/y=w290:dbl)
                      n111 = Subtract(x=w275, y=w273) -> (x-y=w281:dbl)
                      n112 = Multiply(x=w290, y=w281) -> (x*y=w289:dbl)
                      n113 = Bundle By Name(cluster=cluster{"Fs":dbl, "#s":dbl} {"Fs"=1000.0, "#s"=1000.0} ("sampling info"), "Fs"=w283, "#s"=w289) -> (w291:cluster{"Fs":dbl, "#s":dbl})
                      n114 = call <vilib>:"Square Waveform.vi"("duty cycle (%)"=0.0, "offset"=0.0, "sampling info"=w291, "reset signal"=TRUE, "amplitude"=0.0, "frequency"=w284) -> ("signal out"=w279:waveform(dbl))  [unwired: 4 in, 1 out]
                      n115 = local read "一个正弦波形图"() -> (w280:waveform(dbl))
                      n116 = call "拼接信号27"("Input Signal B"=w280, "Input Signal A"=w279) -> ("Appended Signals"=w278:dynamicdata)  [unwired: 8 in, 1 out]
                      n117 = call "拼接信号29"("Input Signal B"=w271, "Input Signal A"=w278) -> ("Appended Signals"=→"中短平+2正弦":dynamicdata)  [unwired: 8 in, 1 out]
                    }
                    frame #3 {
                      n118 = local read "起始偏移（正弦）"() -> (w332:dbl)
                      n119 = Greater Or Equal?(x=w311, y=2.0) -> (x >= y?=w308:bool)
                      n120 = case shown="真" w308 {
                        tunnel: [w358 w363] -> w310
                        tunnel: w311 -> [w357 w362]
                        frame False {
                          n121 = case shown="1, 默认" w357 {
                            tunnel: [w359] -> w358
                            frame 1, Default {
                              n122 = local read "中短平+2正弦"() -> (w360:dynamicdata)
                              n123 = local read "起始平+1正弦"() -> (w361:dynamicdata)
                              n124 = call "拼接信号19"("Input Signal B"=w360, "Input Signal A"=w361) -> ("Appended Signals"=w359:dynamicdata)  [unwired: 8 in, 1 out]
                            }
                          }
                        }
                        frame True {
                          n125 = stacked-sequence {
                            tunnel: [_ _ w372] -> w363
                            tunnel: w362 -> [_ w366 _]
                            frame #0 {
                              n126 = local read "起始平+1正弦"() -> (w364:dynamicdata)
                              n127 = local write "间隔长平+正弦信号"(w364) -> ()
                            }
                            frame #1 {
                              n128 = Decrement(x=w366) -> (x-1=w365:dbl)
                              n129 = for {
                                N: w365 -> [_]
                                n130 = local read "间隔长平+正弦信号"() -> (w369:dynamicdata)
                                n131 = local read "长平+1正弦"() -> (w368:dynamicdata)
                                n132 = call "拼接信号30"("Input Signal B"=w368, "Input Signal A"=w369) -> ("Appended Signals"=w367:dynamicdata)  [unwired: 8 in, 1 out]
                                n133 = local write "间隔长平+正弦信号"(w367) -> ()
                              }
                            }
                            frame #2 {
                              n134 = local read "间隔长平+正弦信号"() -> (w371:dynamicdata)
                              n135 = local read "中短平+2正弦"() -> (w370:dynamicdata)
                              n136 = call "拼接信号31"("Input Signal B"=w370, "Input Signal A"=w371) -> ("Appended Signals"=w372:dynamicdata)  [unwired: 8 in, 1 out]
                            }
                          }
                        }
                      }
                      n137 = Divide(x=w340, y=w339) -> (x/y=w346:dbl)
                      n138 = Multiply(x=w346, y=w332) -> (x*y=w345:dbl)
                      n139 = Bundle By Name(cluster=cluster{"Fs":dbl, "#s":dbl} {"Fs"=1000.0, "#s"=1000.0} ("sampling info"), "Fs"=w340, "#s"=w345) -> (w347:cluster{"Fs":dbl, "#s":dbl})
                      n140 = call <vilib>:"Square Waveform.vi"("duty cycle (%)"=0.0, "offset"=0.0, "sampling info"=w347, "reset signal"=TRUE, "amplitude"=0.0, "frequency"=w339) -> ("signal out"=w333:waveform(dbl))  [unwired: 4 in, 1 out]
                      n141 = local read "长平+1正弦"() -> (w334:dynamicdata)
                      n142 = Subtract(x=w312, y=4.0) -> (x-y=w318:dbl)
                      n143 = Decrement(x=w311) -> (x-1=w317:dbl)
                      n144 = Subtract(x=w318, y=w317) -> (x-y=w315:dbl)
                      n145 = Greater Or Equal?(x=w315, y=1.0) -> (x >= y?=w314:bool)
                      n146 = Decrement(x=w315) -> (x-1=w313:dbl)
                      n147 = call "拼接信号32"("Input Signal B"=w333, "Input Signal A"=w334) -> ("Appended Signals"=w338:dynamicdata)  [unwired: 8 in, 1 out]
                      n148 = case shown="真" w314 {
                        tunnel: w313 -> [_ w350]
                        tunnel: [_ w349] -> w309
                        frame False {
                        }
                        frame True {
                          n149 = stacked-sequence {
                            tunnel: w350 -> [_ w352 _]
                            tunnel: [_ _ w356] -> w349
                            frame #0 {
                              n150 = local read "长平+1正弦"() -> (w351:dynamicdata)
                              n151 = local write "长平组信号正弦"(w351) -> ()
                            }
                            frame #1 {
                              n152 = for {
                                N: w352 -> [_]
                                n153 = local read "长平组信号正弦"() -> (w355:dynamicdata)
                                n154 = local read "长平+1正弦"() -> (w354:dynamicdata)
                                n155 = call "拼接信号33"("Input Signal B"=w354, "Input Signal A"=w355) -> ("Appended Signals"=w353:dynamicdata)  [unwired: 8 in, 1 out]
                                n156 = local write "长平组信号正弦"(w353) -> ()
                              }
                            }
                            frame #2 {
                              n157 = local read "长平组信号正弦"() -> (w356:dynamicdata)
                            }
                          }
                        }
                      }
                      n158 = call "拼接信号34"("Input Signal B"=w309, "Input Signal A"=w310) -> ("Appended Signals"=w337:dynamicdata)  [unwired: 8 in, 1 out]
                      n159 = Bundle By Name("Y"=dbl[] []) -> (w326:waveform(dbl))  [unwired: 1 in]
                      n160 = call "拼接信号35"("Input Signal B"=w338, "Input Signal A"=w337) -> ("Appended Signals"=w324:dynamicdata)  [unwired: 8 in, 1 out]
                      n161 = case shown="真" w321 {
                        tunnel: [w373 w375] -> w323
                        tunnel: w324 -> [w373 w374]
                        frame False {
                        }
                        frame True {
                          n162 = Negate(x=w374) -> (-x=w375:dynamicdata)
                        }
                      }
                      n163 = Divide(x=w327, y=2.0) -> (x/y=w335:dbl)
                      n164 = Add(x=w335, y=w323) -> (x+y=w322:dynamicdata)
                      n165 = case shown="2, 默认" w331 {
                        tunnel: w322 -> [w377 w380]
                        tunnel: [w377 w380] -> w330
                        tunnel: [w376 w381] -> w328
                        tunnel: w327 -> [_ w379]
                        tunnel: w326 -> [w376 w378]
                        tunnel: [w376 w378] -> w325
                        frame 1 {
                        }
                        frame 2, Default {
                          n166 = Negate(x=w380) -> (-x=w382:dynamicdata)
                          n167 = Add(x=w382, y=w379) -> (x+y=w381:dynamicdata)
                        }
                      }
                    }
                  }
                }
                frame 1 {
                  n168 = Not Equal?(x=w387, y=1.0) -> (x != y?=w386:bool)
                  n169 = case shown="真" w386 {
                    tunnel: w398 -> [w407 w451]
                    tunnel: w397 -> [w419 w450]
                    tunnel: w396 -> [_ w449]
                    tunnel: w395 -> [w399 w448]
                    tunnel: [w417 w447] -> w394
                    tunnel: w393 -> [w420 w446]
                    tunnel: [w415 w445] -> w392
                    tunnel: [w415 w444] -> w391
                    tunnel: w390 -> [_ w443]
                    tunnel: w389 -> [w414 w442]
                    tunnel: w387 -> [w403 w441]
                    tunnel: w385 -> [_ w440]
                    tunnel: w384 -> [_ w439]
                    tunnel: w383 -> [_ w438]
                    frame False {
                      n170 = Divide(x=w399, y=2.0) -> (x/y=w400:dbl)
                      n171 = Divide(x=w419, y=w407) -> (x/y=w423:dbl)
                      n172 = Divide(x=w419, y=w407) -> (x/y=w404:dbl)
                      n173 = Multiply(x=w423, y=w420) -> (x*y=w422:dbl)
                      n174 = Bundle By Name(cluster=cluster{"Fs":dbl, "#s":dbl} {"Fs"=1000.0, "#s"=1000.0} ("sampling info"), "Fs"=w419, "#s"=w422) -> (w428:cluster{"Fs":dbl, "#s":dbl})
                      n175 = Multiply(x=w404, y=w403) -> (x*y=w405:dbl)
                      n176 = Bundle By Name(cluster=cluster{"Fs":dbl, "#s":dbl} {"Fs"=1000.0, "#s"=1000.0} ("sampling info"), "Fs"=w419, "#s"=w405) -> (w412:cluster{"Fs":dbl, "#s":dbl})
                      n177 = call <vilib>:"Square Waveform.vi"("duty cycle (%)"=50.0, "offset"=0.0, "sampling info"=w428, "reset signal"=TRUE, "amplitude"=w400, "frequency"=w407) -> ("signal out"=w421:waveform(dbl))  [unwired: 4 in, 1 out]
                      n178 = call <vilib>:"Square Waveform.vi"("duty cycle (%)"=0.0, "offset"=0.0, "sampling info"=w412, "reset signal"=TRUE, "amplitude"=0.0, "frequency"=w407) -> ("signal out"=w408:waveform(dbl))  [unwired: 4 in, 1 out]
                      n179 = case shown="真" w414 {
                        tunnel: w421 -> [w435 w437]
                        tunnel: [w435 w436] -> w402
                        frame False {
                        }
                        frame True {
                          n180 = Negate(x=w437) -> (-x=w436:waveform(dbl))
                        }
                      }
                      n181 = case shown="真" w414 {
                        tunnel: w408 -> [w430 w434]
                        tunnel: [w430 w433] -> w418
                        tunnel: w399 -> [_ w431]
                        frame False {
                        }
                        frame True {
                          n182 = Negate(x=w434) -> (-x=w432:waveform(dbl))
                          n183 = Add(x=w431, y=w432) -> (x+y=w433:waveform(dbl))
                        }
                      }
                      n184 = Add(x=w400, y=w402) -> (x+y=w401:waveform(dbl))
                      n185 = Bundle By Name("Y"=dbl[] []) -> (w415:waveform(dbl))  [unwired: 1 in]
                      n186 = call "拼接信号38"("Input Signal B"=w418, "Input Signal A"=w401) -> ("Appended Signals"=w417:dynamicdata)  [unwired: 8 in, 1 out]
                    }
                    frame True {
                      n187 = stacked-sequence {
                        tunnel: w451 -> [w456 w515 w525 w539 w597]
                        tunnel: w450 -> [w474 w514 w524 w540 w596]
                        tunnel: w449 -> [_ w517 _ _ _]
                        tunnel: w448 -> [w473 w516 w521 w549 w598]
                        tunnel: [_ _ _ _ w587] -> w447
                        tunnel: w446 -> [_ w513 _ _ w575]
                        tunnel: [_ _ _ _ w584] -> w445
                        tunnel: [_ _ _ _ w583] -> w444
                        tunnel: w441 -> [w453 w500 _ w538 _]
                        tunnel: w443 -> [_ _ _ _ w576]
                        tunnel: w442 -> [_ _ _ _ w579]
                        tunnel: w440 -> [_ _ _ w536 _]
                        tunnel: w439 -> [_ w493 w518 _ _]
                        tunnel: w438 -> [_ _ _ _ w572]
                        frame #0 {
                          n188 = Divide(x=w473, y=2.0) -> (x/y=w457:dbl)
                          n189 = Greater?(x=w453, y=2.0) -> (0:w452:bool)
                          n190 = Divide(x=w474, y=w456) -> (x/y=w455:dbl)
                          n191 = case shown="真" w452 {
                            tunnel: w474 -> [_ w488]
                            tunnel: [_ w484] -> w464
                            tunnel: w457 -> [_ w481]
                            tunnel: w456 -> [_ w480]
                            tunnel: w455 -> [_ w478]
                            tunnel: w453 -> [_ w475]
                            frame False {
                            }
                            frame True {
                              n192 = Subtract(x=w475, y=2.0) -> (x-y=w477:dbl)
                              n193 = Multiply(x=w478, y=w477) -> (x*y=w479:dbl)
                              n194 = Bundle By Name(cluster=cluster{"Fs":dbl, "#s":dbl} {"Fs"=1000.0, "#s"=1000.0} ("sampling info"), "Fs"=w488, "#s"=w479) -> (w486:cluster{"Fs":dbl, "#s":dbl})
                              n195 = call <vilib>:"Square Waveform.vi"("duty cycle (%)"=100.0, "offset"=0.0, "sampling info"=w486, "reset signal"=TRUE, "amplitude"=w481, "frequency"=w480) -> ("signal out"=w484:waveform(dbl))  [unwired: 4 in, 1 out]
                            }
                          }
                          n196 = Bundle By Name(cluster=cluster{"Fs":dbl, "#s":dbl} {"Fs"=1000.0, "#s"=1000.0} ("sampling info"), "Fs"=w474, "#s"=w455) -> (w471:cluster{"Fs":dbl, "#s":dbl})
                          n197 = call <vilib>:"Square Waveform.vi"("duty cycle (%)"=50.0, "offset"=0.0, "sampling info"=w471, "reset signal"=TRUE, "amplitude"=w457, "frequency"=w456) -> ("signal out"=w462:waveform(dbl))  [unwired: 4 in, 1 out]
                          n198 = call "从动态数据转换2"("Dynamic Data Type"=w462) -> ("Array"=w469:dbl[])  [unwired: 3 in]
                          n199 = Unbundle By Name(w462) -> ("t0"=w467:timestamp, "dt"=w468:dbl)  [unwired: 1 out]
                          n200 = Reverse 1D Array(array=w469) -> (reversed array=w470:dbl[])
                          n201 = Bundle By Name("Y"=w470, "t0"=w467, "dt"=w468) -> (w465:waveform(dbl))  [unwired: 1 in]
                          n202 = case shown="3, 默认" w453 {
                            tunnel: w465 -> [w491 w492]
                            tunnel: w464 -> [w490 _]
                            tunnel: [w489 w492] -> w463
                            frame 3, Default {
                              n203 = call "拼接信号5"("Input Signal B"=w490, "Input Signal A"=w491) -> ("Appended Signals"=w489:dynamicdata)  [unwired: 8 in, 1 out]
                            }
                            frame 2 {
                            }
                          }
                          n204 = call "拼接信号6"("Input Signal B"=w462, "Input Signal A"=w463) -> ("Appended Signals"=→"一个凸起波形图":dynamicdata)  [unwired: 8 in, 1 out]
                        }
                        frame #1 {
                          n205 = Decrement(x=w513) -> (x-1=w494:dbl)
                          n206 = Multiply(x=w517, y=2.0) -> (x*y=w499:dbl)
                          n207 = Multiply(x=w500, y=w494) -> (x*y=w498:dbl)
                          n208 = Subtract(x=w499, y=w498) -> (x-y=w496:dbl)
                          n209 = Divide(x=w516, y=2.0) -> (x/y=w502:dbl)
                          n210 = Divide(x=w514, y=w515) -> (x/y=w510:dbl)
                          n211 = Divide(x=w496, y=w494) -> (x/y=w495:dbl)
                          n212 = Subtract(x=w495, y=w493) -> (x-y=w504:dbl)
                          "起始水平线个数（方波）" <- w504
                          n213 = Multiply(x=w510, y=w504) -> (x*y=w509:dbl)
                          n214 = Bundle By Name(cluster=cluster{"Fs":dbl, "#s":dbl} {"Fs"=1000.0, "#s"=1000.0} ("sampling info"), "Fs"=w514, "#s"=w509) -> (w511:cluster{"Fs":dbl, "#s":dbl})
                          n215 = call <vilib>:"Square Waveform.vi"("duty cycle (%)"=0.0, "sampling info"=w511, "reset signal"=TRUE, "amplitude"=w502, "frequency"=w515) -> ("signal out"=w508:waveform(dbl))  [unwired: 5 in, 1 out]
                          n216 = local read "一个凸起波形图"() -> (w507:dynamicdata)
                          n217 = call "拼接信号8"("Input Signal B"=w507, "Input Signal A"=w508) -> ("Appended Signals"=→"起始平+1凸":dynamicdata)  [unwired: 8 in, 1 out]
                          "起始偏移（方波）" <- w493
                        }
                        frame #2 {
                          n218 = local read "起始水平线个数（方波）"() -> (w526:dbl)
                          n219 = Divide(x=w521, y=2.0) -> (x/y=w519:dbl)
                          n220 = Add(x=w518, y=w526) -> (x+y=w527:dbl)
                          "长水平线数量（方波）" <- w527
                          n221 = Divide(x=w524, y=w525) -> (x/y=w533:dbl)
                          n222 = Multiply(x=w533, y=w527) -> (x*y=w532:dbl)
                          n223 = Bundle By Name(cluster=cluster{"Fs":dbl, "#s":dbl} {"Fs"=1000.0, "#s"=1000.0} ("sampling info"), "Fs"=w524, "#s"=w532) -> (w534:cluster{"Fs":dbl, "#s":dbl})
                          n224 = local read "一个凸起波形图"() -> (w528:dynamicdata)
                          n225 = call <vilib>:"Square Waveform.vi"("duty cycle (%)"=0.0, "offset"=0.0, "sampling info"=w534, "reset signal"=TRUE, "amplitude"=w519, "frequency"=w525) -> ("signal out"=w529:waveform(dbl))  [unwired: 4 in, 1 out]
                          n226 = call "拼接信号22"("Input Signal B"=w528, "Input Signal A"=w529) -> ("Appended Signals"=→"长平+1凸":dynamicdata)  [unwired: 8 in, 1 out]
                        }
                        frame #3 {
                          n227 = local read "长水平线数量（方波）"() -> (w542:dbl)
                          n228 = Divide(x=w549, y=2.0) -> (x/y=w548:dbl)
                          n229 = Subtract(x=w542, y=w538) -> (x-y=w537:dbl)
                          n230 = Subtract(x=w537, y=w536) -> (x-y=w557:dbl)
                          n231 = Divide(x=w540, y=w539) -> (x/y=w541:dbl)
                          n232 = Multiply(x=w541, y=w557) -> (x*y=w562:dbl)
                          n233 = Multiply(x=w541, y=w536) -> (x*y=w553:dbl)
                          n234 = Bundle By Name(cluster=cluster{"Fs":dbl, "#s":dbl} {"Fs"=1000.0, "#s"=1000.0} ("sampling info"), "Fs"=w540, "#s"=w562) -> (w564:cluster{"Fs":dbl, "#s":dbl})
                          n235 = Bundle By Name(cluster=cluster{"Fs":dbl, "#s":dbl} {"Fs"=1000.0, "#s"=1000.0} ("sampling info"), "Fs"=w540, "#s"=w553) -> (w555:cluster{"Fs":dbl, "#s":dbl})
                          n236 = call <vilib>:"Square Waveform.vi"("duty cycle (%)"=0.0, "offset"=0.0, "sampling info"=w555, "reset signal"=TRUE, "amplitude"=w548, "frequency"=w539) -> ("signal out"=w543:waveform(dbl))  [unwired: 4 in, 1 out]
                          n237 = call <vilib>:"Square Waveform.vi"("duty cycle (%)"=0.0, "offset"=0.0, "sampling info"=w564, "reset signal"=TRUE, "amplitude"=w548, "frequency"=w539) -> ("signal out"=w561:waveform(dbl))  [unwired: 4 in, 1 out]
                          n238 = local read "一个凸起波形图"() -> (w560:dynamicdata)
                          n239 = local read "一个凸起波形图"() -> (w547:dynamicdata)
                          n240 = call "拼接信号11"("Input Signal B"=w560, "Input Signal A"=w561) -> ("Appended Signals"=w546:dynamicdata)  [unwired: 8 in, 1 out]
                          n241 = call "拼接信号12"("Input Signal B"=w547, "Input Signal A"=w543) -> ("Appended Signals"=w545:dynamicdata)  [unwired: 8 in, 1 out]
                          n242 = call "拼接信号10"("Input Signal B"=w545, "Input Signal A"=w546) -> ("Appended Signals"=→"中、短平+2凸":dynamicdata)  [unwired: 8 in, 1 out]
                        }
                        frame #4 {
                          n243 = local read "起始偏移（方波）"() -> (w582:dbl)
                          n244 = Divide(x=w598, y=2.0) -> (x/y=w594:dbl)
                          n245 = Divide(x=w596, y=w597) -> (x/y=w603:dbl)
                          n246 = Greater Or Equal?(x=w572, y=2.0) -> (x >= y?=w577:bool)
                          n247 = Multiply(x=w603, y=w582) -> (x*y=w602:dbl)
                          n248 = case shown="真" w577 {
                            tunnel: [w615 w620] -> w591
                            tunnel: w572 -> [w614 w619]
                            frame False {
                              n249 = case shown="1, 默认" w614 {
                                tunnel: [w616] -> w615
                                frame 1, Default {
                                n250 = local read "中、短平+2凸"() -> (w617:dynamicdata)
                                n251 = local read "起始平+1凸"() -> (w618:dynamicdata)
                                n252 = call "拼接信号4"("Input Signal B"=w617, "Input Signal A"=w618) -> ("Appended Signals"=w616:dynamicdata)  [unwired: 8 in, 1 out]
                                }
                              }
                            }
                            frame True {
                              n253 = stacked-sequence {
                                tunnel: [_ _ w629] -> w620
                                tunnel: w619 -> [_ w623 _]
                                frame #0 {
                                n254 = local read "起始平+1凸"() -> (w621:dynamicdata)
                                n255 = local write "间隔长平+凸信号"(w621) -> ()
                                }
                                frame #1 {
                                n256 = Decrement(x=w623) -> (x-1=w622:dbl)
                                n257 = for {
                                N: w622 -> [_]
                                n258 = local read "间隔长平+凸信号"() -> (w626:dynamicdata)
                                n259 = local read "长平+1凸"() -> (w625:dynamicdata)
                                n260 = call "拼接信号7"("Input Signal B"=w625, "Input Signal A"=w626) -> ("Appended Signals"=w624:dynamicdata)  [unwired: 8 in, 1 out]
                                n261 = local write "间隔长平+凸信号"(w624) -> ()
                                }
                                }
                                frame #2 {
                                n262 = local read "间隔长平+凸信号"() -> (w628:dynamicdata)
                                n263 = local read "中、短平+2凸"() -> (w627:dynamicdata)
                                n264 = call "拼接信号9"("Input Signal B"=w627, "Input Signal A"=w628) -> ("Appended Signals"=w629:dynamicdata)  [unwired: 8 in, 1 out]
                                }
                              }
                            }
                          }
                          n265 = Bundle By Name(cluster=cluster{"Fs":dbl, "#s":dbl} {"Fs"=1000.0, "#s"=1000.0} ("sampling info"), "Fs"=w596, "#s"=w602) -> (w604:cluster{"Fs":dbl, "#s":dbl})
                          n266 = call <vilib>:"Square Waveform.vi"("duty cycle (%)"=0.0, "offset"=0.0, "sampling info"=w604, "reset signal"=TRUE, "amplitude"=w594, "frequency"=w597) -> ("signal out"=w592:waveform(dbl))  [unwired: 4 in, 1 out]
                          n267 = local read "长平+1凸"() -> (w593:dynamicdata)
                          n268 = call "拼接信号14"("Input Signal B"=w592, "Input Signal A"=w593) -> ("Appended Signals"=w589:dynamicdata)  [unwired: 8 in, 1 out]
                          n269 = Subtract(x=w575, y=4.0) -> (x-y=w573:dbl)
                          n270 = Decrement(x=w572) -> (x-1=w571:dbl)
                          n271 = Subtract(x=w573, y=w571) -> (x-y=w567:dbl)
                          n272 = Decrement(x=w567) -> (x-1=w568:dbl)
                          n273 = Greater Or Equal?(x=w567, y=1.0) -> (x >= y?=w569:bool)
                          n274 = case shown="真" w569 {
                            tunnel: w568 -> [_ w607]
                            tunnel: [_ w606] -> w566
                            frame False {
                            }
                            frame True {
                              n275 = stacked-sequence {
                                tunnel: w607 -> [_ w609 _]
                                tunnel: [_ _ w613] -> w606
                                frame #0 {
                                n276 = local read "长平+1凸"() -> (w608:dynamicdata)
                                n277 = local write "长平组信号"(w608) -> ()
                                }
                                frame #1 {
                                n278 = for {
                                N: w609 -> [_]
                                n279 = local read "长平组信号"() -> (w612:dynamicdata)
                                n280 = local read "长平+1凸"() -> (w611:dynamicdata)
                                n281 = call "拼接信号13"("Input Signal B"=w611, "Input Signal A"=w612) -> ("Appended Signals"=w610:dynamicdata)  [unwired: 8 in, 1 out]
                                n282 = local write "长平组信号"(w610) -> ()
                                }
                                }
                                frame #2 {
                                n283 = local read "长平组信号"() -> (w613:dynamicdata)
                                }
                              }
                            }
                          }
                          n284 = call "拼接信号20"("Input Signal B"=w566, "Input Signal A"=w591) -> ("Appended Signals"=w590:dynamicdata)  [unwired: 8 in, 1 out]
                          n285 = call "拼接信号21"("Input Signal B"=w589, "Input Signal A"=w590) -> ("Appended Signals"=w581:dynamicdata)  [unwired: 8 in, 1 out]
                          n286 = case shown="真" w579 {
                            tunnel: w581 -> [w630 w632]
                            tunnel: [w630 w631] -> w580
                            frame False {
                            }
                            frame True {
                              n287 = Negate(x=w632) -> (-x=w631:dynamicdata)
                            }
                          }
                          n288 = Add(x=w594, y=w580) -> (x+y=w588:dynamicdata)
                          n289 = Bundle By Name("Y"=dbl[] []) -> (w585:waveform(dbl))  [unwired: 1 in]
                          n290 = case shown="1, 默认" w576 {
                            tunnel: w588 -> [w634 _]
                            tunnel: [w634 w635] -> w587
                            tunnel: w585 -> [w633 w635]
                            tunnel: [w633 w635] -> w584
                            tunnel: [w633 w635] -> w583
                            frame 1, Default {
                            }
                            frame 0 {
                            }
                          }
                        }
                      }
                    }
                  }
                }
                frame 2 {
                  n291 = Equal?(x=w651, y=1) -> (x = y?=w648:bool)
                  n292 = Equal?(x=w636, y=2) -> (x = y?=w647:bool)
                  n293 = local read "1波形图"() -> (w645:waveform(dbl))
                  n294 = local read "5波形图"() -> (w638:waveform(dbl))
                  n295 = local read "6波形图"() -> (w637:waveform(dbl))
                  n296 = Bundle By Name("Y"=dbl[] []) -> (w642:waveform(dbl))  [unwired: 1 in]
                  n297 = And(x=w648, y=w647) -> (x .and. y?=w646:bool)
                  n298 = case shown="假" w646 {
                    tunnel: w645 -> [_ w673]
                    tunnel: [w652 w673] -> w644
                    tunnel: w642 -> [w656 w672]
                    tunnel: [w654 w672] -> w641
                    tunnel: [w653 w672] -> w640
                    tunnel: w639 -> [w660 _]
                    tunnel: w638 -> [w658 _]
                    tunnel: w637 -> [w657 _]
                    tunnel: w636 -> [w655 _]
                    frame False {
                      n299 = Equal To 0?(x=w660) -> (x = 0?=w659:bool)
                      n300 = case shown="真" w659 {
                        tunnel: w658 -> [_ w662]
                        tunnel: w657 -> [_ w661]
                        tunnel: w656 -> [_ w666]
                        tunnel: w655 -> [_ w667]
                        tunnel: [_ w665] -> w654
                        tunnel: [_ w664] -> w653
                        tunnel: [_ w663] -> w652
                        frame False {
                        }
                        frame True {
                          n301 = case shown="4" w667 {
                            tunnel: [w668 w669] -> w665
                            tunnel: w666 -> [w668 w671]
                            tunnel: [w668 w670] -> w664
                            tunnel: [w668 w671] -> w663
                            tunnel: w662 -> [_ w670]
                            tunnel: w661 -> [_ w669]
                            frame 2, Default {
                            }
                            frame 4 {
                            }
                          }
                        }
                      }
                    }
                    frame True {
                    }
                  }
                }
              }
              "ME Channel 3" <- w6
              "ME Channel 4" <- w20
              "Hall Channel 1" <- w4
              n302 = case shown="1" w70 {
                tunnel: w72 -> [w688 w972 _]
                tunnel: "Speed FM" -> [w687 w973 _]
                tunnel: w69 -> [w686 w975 _]
                tunnel: "波形发生率Fs" -> [w685 w974 _]
                tunnel: w68 -> [w684 w971 _]
                tunnel: [w677 w970 w1066] -> w8
                tunnel: w65 -> [w683 w966 _]
                tunnel: w66 -> [w682 _ _]
                tunnel: w67 -> [w681 w968 _]
                tunnel: w66 -> [w680 w967 _]
                tunnel: [w679 w969 w1066] -> w12
                tunnel: [w678 w965 w1066] -> w21
                tunnel: [w676 w963 0.0] -> w25
                tunnel: w11 -> [w674 w964 _]
                tunnel: w30 -> [w675 _ _]
                tunnel: [_ w962 _] -> w7
                frame 0, Default {
                  n303 = stacked-sequence "层叠式顺序结构" {
                    tunnel: w688 -> [w695 _ _ _ w855]
                    tunnel: w687 -> [w689 w724 w753 w799 w857]
                    tunnel: w686 -> [w707 w723 _ w797 w856]
                    tunnel: w685 -> [w694 w725 w754 w800 w858]
                    tunnel: w684 -> [w706 _ _ w798 w853]
                    tunnel: w683 -> [_ w721 w752 w802 w850]
                    tunnel: w682 -> [w693 _ _ _ _]
                    tunnel: w681 -> [_ _ _ _ w852]
                    tunnel: w680 -> [_ _ _ _ _]
                    tunnel: [_ _ _ _ w865] -> w679
                    tunnel: [_ _ _ _ w863] -> w678
                    tunnel: [_ _ _ _ w859] -> w677
                    tunnel: [w690 _ _ _ _] -> w676
                    tunnel: w675 -> [_ _ _ _ w847]
                    tunnel: w674 -> [_ _ _ _ w843]
                    frame #0 {
                      n304 = Equal To 0?(x=w689) -> (x = 0?=w692:bool)
                      n305 = Divide(x=w694, y=w689) -> (x/y=w701:dbl)
                      n306 = case shown="真" w692 {
                        tunnel: w689 -> [w715 _]
                        tunnel: w693 -> [w713 _]
                        tunnel: [w709 0.0] -> w691
                        frame False {
                          n307 = Reciprocal(x=w715) -> (1/x=w714:dbl)
                          n308 = Multiply(x=w713, y=w714) -> (x*y=w712:dbl)
                          n309 = Reciprocal(x=w712) -> (1/x=w711:dbl)
                          n310 = Multiply(x=w711, y=60.0) -> (x*y=w709:dbl)
                        }
                        frame True {
                        }
                      }
                      n311 = Divide(x=w707, y=2.0) -> (x/y=w696:dbl)
                      "曲轴正弦偏移量" <- w696
                      n312 = Multiply(x=w701, y=w695) -> (x*y=w704:dbl)
                      n313 = Bundle By Name(cluster=cluster{"Fs":dbl, "#s":dbl} {"Fs"=1000.0, "#s"=1000.0} ("sampling info"), "Fs"=w694, "#s"=w704) -> (w705:cluster{"Fs":dbl, "#s":dbl})
                      n314 = call <vilib>:"Sine Waveform.vi"("offset"=0.0, "sampling info"=w705, "reset signal"=TRUE, "amplitude"=w696, "frequency"=w689) -> ("signal out"=w703:waveform(dbl))  [unwired: 5 in, 1 out]
                      n315 = case shown="真" w706 {
                        tunnel: w703 -> [w718 w719]
                        tunnel: [w717 w719] -> w702
                        frame False {
                          n316 = Negate(x=w718) -> (-x=w717:waveform(dbl))
                        }
                        frame True {
                        }
                      }
                      n317 = Round To Nearest(number=w691) -> (nearest integer value=w690:dbl)
                      n318 = Add(x=w696, y=w702) -> (x+y=→"曲轴正弦波形图":waveform(dbl))
                    }
                    frame #1 {
                      n319 = Equal To 0?(x=w721) -> (x = 0?=w720:bool)
                      n320 = Not(x=w720) -> (.not. x?=w722:bool)
                      n321 = case shown="真" w722 {
                        tunnel: w725 -> [_ w730]
                        tunnel: w724 -> [_ w729]
                        tunnel: w723 -> [_ w726]
                        frame False {
                        }
                        frame True {
                          n322 = Divide(x=w730, y=w729) -> (x/y=w728:dbl)
                          n323 = Multiply(x=0.4, y=w728) -> (x*y=w733:dbl)
                          n324 = Divide(x=w726, y=2.0) -> (x/y=w727:dbl)
                          n325 = Bundle By Name(cluster=cluster{"Fs":dbl, "#s":dbl} {"Fs"=1000.0, "#s"=1000.0} ("sampling info"), "Fs"=w730, "#s"=w733) -> (w749:cluster{"Fs":dbl, "#s":dbl})
                          n326 = Multiply(x=0.3, y=w728) -> (x*y=w739:dbl)
                          "圆弧点数" <- w739
                          n327 = call <vilib>:"Sine Waveform.vi"("offset"=0.0, "sampling info"=w749, "reset signal"=TRUE, "amplitude"=w727, "frequency"=w729) -> ("signal out"=w744:waveform(dbl))  [unwired: 5 in, 1 out]
                          "部分\n正弦\n波形图" <- w744
                          n328 = To Long Integer(number=w739) -> (32bit integer=w742:i32)
                          n329 = Unbundle By Name(w744) -> ("t0"=→"t0":timestamp, "dt"=→"dt":dbl, "Y"=w745:dbl[])
                          n330 = Increment(x=w742) -> (x+1=→"循环次数":i32)
                          n331 = Array Size(array=w745) -> (size(s)=w747:i32)
                          n332 = Decrement(x=w747) -> (x-1=w746:i32)
                          n333 = Index Array(array=w745, index=w746) -> (element=w740:dbl)
                          "圆半径" <- w740
                          n334 = Divide(x=w740, y=w739) -> (x/y=→"x轴取点间隔":dbl)
                        }
                      }
                    }
                    frame #2 {
                      n335 = Equal To 0?(x=w752) -> (x = 0?=w751:bool)
                      n336 = Not(x=w751) -> (.not. x?=w750:bool)
                      n337 = case shown="真" w750 {
                        tunnel: w754 -> [_ w759]
                        tunnel: w753 -> [_ w758]
                        tunnel: w752 -> [_ w755]
                        frame False {
                        }
                        frame True {
                          n338 = local read "循环次数"() -> (w781:i32)
                          n339 = Increment(x=w755) -> (x+1=w762:dbl)
                          n340 = Divide(x=w762, y=2.0) -> (x/y=w761:dbl)
                          n341 = for {
                            N: w781 -> [_]
                            tunnel: [w792] -> w780 mode=indexing
                            i -> [w793]
                            n342 = local read "x轴取点间隔"() -> (w794:dbl)
                            n343 = Multiply(x=w794, y=w793) -> (x*y=w795:dbl)
                            n344 = Add(x=0.0, y=w795) -> (x+y=w792:dbl)
                          }
                          n345 = Subtract(x=w761, y=0.7) -> (x-y=w756:dbl)
                          n346 = local read "圆半径"() -> (w782:dbl)
                          n347 = Divide(x=w759, y=w758) -> (x/y=w757:dbl)
                          n348 = Multiply(x=w757, y=w756) -> (x*y=w774:dbl)
                          n349 = Multiply(x=2.0, y=w782) -> (x*y=w790:dbl)
                          n350 = Bundle By Name(cluster=cluster{"Fs":dbl, "#s":dbl} {"Fs"=1000.0, "#s"=1000.0} ("sampling info"), "Fs"=w759, "#s"=w774) -> (w775:cluster{"Fs":dbl, "#s":dbl})
                          n351 = Square(x=w780) -> (x^2=w788:dbl[])
                          n352 = Multiply(x=w780, y=w790) -> (x*y=w789:dbl[])
                          n353 = call <vilib>:"Square Waveform.vi"("duty cycle (%)"=0.0, "offset"=0.0, "sampling info"=w775, "reset signal"=TRUE, "amplitude"=0.0, "frequency"=w758) -> ("signal out"=w773:waveform(dbl))  [unwired: 4 in, 1 out]
                          n354 = Subtract(x=w789, y=w788) -> (x-y=w787:dbl[])
                          n355 = Square Root(x=w787) -> (sqrt(x)=w786:dbl[])
                          n356 = Subtract(x=w782, y=w786) -> (x-y=w785:dbl[])
                          n357 = local read "t0"() -> (w772:timestamp)
                          n358 = local read "dt"() -> (w771:dbl)
                          n359 = Bundle By Name("Y"=w773, "t0"=w772, "dt"=w771) -> (w769:waveform(dbl))  [unwired: 1 in]
                          "半\n缺\n齿\n水\n平\n线" <- w769
                          n360 = local read "部分\n正弦\n波形图"() -> (w768:waveform(dbl))
                          n361 = Delete From Array(array=w785, length=1 ("索引"), index=0 ("长度")) -> (array with subset deleted=w779:dbl[])  [unwired: 1 out]
                          n362 = Bundle By Name("Y"=w779, "t0"=w772, "dt"=w771) -> (w770:waveform(dbl))  [unwired: 1 in]
                          "圆\n弧" <- w770
                          n363 = call "拼接信号"("Input Signal B"=w769, "Input Signal A"=w770) -> ("Appended Signals"=w767:dynamicdata)  [unwired: 8 in, 1 out]
                          "圆\n弧\n+\n水\n平" <- w767
                          n364 = call "拼接信号2"("Input Signal B"=w767, "Input Signal A"=w768) -> ("Appended Signals"=→"未\n翻\n转\n半\n缺\n齿":dynamicdata)  [unwired: 8 in, 1 out]
                        }
                      }
                    }
                    frame #3 {
                      n365 = Equal To 0?(x=w802) -> (x = 0?=w801:bool)
                      n366 = Not(x=w801) -> (.not. x?=w803:bool)
                      n367 = case shown="真" w803 {
                        tunnel: [w814 w827] -> w804
                        tunnel: w797 -> [w811 _]
                        tunnel: w800 -> [w810 _]
                        tunnel: w799 -> [w805 _]
                        tunnel: w798 -> [w809 w826]
                        frame False {
                          n368 = Multiply(x=w805, y=2.0) -> (x*y=w807:dbl)
                          n369 = Divide(x=w810, y=w807) -> (x/y=w819:dbl)
                          n370 = Multiply(x=w819, y=2.0) -> (x*y=w821:dbl)
                          n371 = Divide(x=w811, y=2.0) -> (x/y=w812:dbl)
                          n372 = Bundle By Name(cluster=cluster{"Fs":dbl, "#s":dbl} {"Fs"=1000.0, "#s"=1000.0} ("sampling info"), "Fs"=w810, "#s"=w821) -> (w822:cluster{"Fs":dbl, "#s":dbl})
                          n373 = call <vilib>:"Sine Waveform.vi"("offset"=0.0, "sampling info"=w822, "reset signal"=TRUE, "amplitude"=w812, "frequency"=w807) -> ("signal out"=w820:waveform(dbl))  [unwired: 5 in, 1 out]
                          n374 = case shown="真" w809 {
                            tunnel: w820 -> [w824 w825]
                            tunnel: [w823 w825] -> w813
                            frame False {
                              n375 = Negate(x=w824) -> (-x=w823:waveform(dbl))
                            }
                            frame True {
                            }
                          }
                          n376 = Add(x=w812, y=w813) -> (x+y=w814:waveform(dbl))
                        }
                        frame True {
                          n377 = local read "未\n翻\n转\n半\n缺\n齿"() -> (w837:dynamicdata)
                          n378 = call "从动态数据转换"("Dynamic Data Type"=w837) -> ("Array"=w836:dbl[])  [unwired: 3 in]
                          n379 = local read "t0"() -> (w834:timestamp)
                          n380 = local read "dt"() -> (w833:dbl)
                          n381 = Reverse 1D Array(array=w836) -> (reversed array=w835:dbl[])
                          n382 = Negate(x=w836) -> (-x=w838:dbl[])
                          n383 = Bundle By Name("Y"=w835, "t0"=w834, "dt"=w833) -> (w831:waveform(dbl))  [unwired: 1 in]
                          n384 = Bundle By Name("Y"=w838, "t0"=w834, "dt"=w833) -> (w832:waveform(dbl))  [unwired: 1 in]
                          n385 = call "拼接信号3"("Input Signal B"=w831, "Input Signal A"=w832) -> ("Appended Signals"=w829:dynamicdata)  [unwired: 8 in, 1 out]
                          n386 = local read "曲轴正弦偏移量"() -> (w830:dbl)
                          n387 = case shown="假" w826 {
                            tunnel: w829 -> [w839 w841]
                            tunnel: [w839 w840] -> w828
                            frame False {
                            }
                            frame True {
                              n388 = Negate(x=w841) -> (-x=w840:dynamicdata)
                            }
                          }
                          n389 = Add(x=w830, y=w828) -> (x+y=w827:dynamicdata)
                        }
                      }
                      "完\n整\n缺\n齿\n波" <- w804
                    }
                    frame #4 {
                      n390 = local read "曲轴正弦波形图"() -> (w867:waveform(dbl))
                      n391 = Not Equal To 0?(x=w850) -> (x != 0?=w848:bool)
                      n392 = local read "完\n整\n缺\n齿\n波"() -> (w866:waveform(dbl))
                      n393 = Equal?(x=w852, y=4.0) -> (x = y?=w849:bool)
                      n394 = call "曲-缺"("Input Signal B"=w866, "Input Signal A"=w867) -> ("Appended Signals"=w845:dynamicdata)  [unwired: 8 in, 1 out]
                      "曲轴" <- w845
                      n395 = Greater Than 0?(x=w843) -> (x > 0?=w846:bool)
                      n396 = Decrement(x=w843) -> (x-1=w842:dbl)
                      n397 = case shown="真" w849 {
                        tunnel: w858 -> [_ w886]
                        tunnel: w857 -> [_ w885]
                        tunnel: w856 -> [_ w884]
                        tunnel: w855 -> [_ w883]
                        tunnel: [_ w882] -> w854
                        tunnel: w853 -> [_ w881]
                        tunnel: w848 -> [_ w880]
                        tunnel: w845 -> [_ w879]
                        tunnel: w847 -> [_ w878]
                        frame False {
                        }
                        frame True {
                          n398 = case shown="真" w880 {
                            tunnel: w886 -> [_ w898]
                            tunnel: w885 -> [_ w897]
                            tunnel: w884 -> [_ w895]
                            tunnel: w883 -> [_ w893]
                            tunnel: [w887 w892] -> w882
                            tunnel: w881 -> [_ w891]
                            tunnel: w879 -> [w887 _]
                            tunnel: w878 -> [_ w888]
                            frame False {
                            }
                            frame True {
                              n399 = stacked-sequence {
                                tunnel: w898 -> [w907 w929]
                                tunnel: w897 -> [w908 w930]
                                tunnel: [_ w924] -> w896
                                tunnel: w895 -> [w909 w921]
                                tunnel: w893 -> [w906 _]
                                tunnel: w891 -> [w904 w928]
                                tunnel: [_ w923] -> w890
                                tunnel: [w900 _] -> w889
                                tunnel: w888 -> [w899 w920]
                                frame #0 {
                                n400 = Subtract(x=w906, y=w899) -> (x-y=w905:dbl)
                                n401 = Divide(x=w907, y=w908) -> (x/y=w914:dbl)
                                n402 = Multiply(x=w914, y=w905) -> (x*y=w915:dbl)
                                n403 = Divide(x=w909, y=2.0) -> (x/y=w901:dbl)
                                n404 = Bundle By Name(cluster=cluster{"Fs":dbl, "#s":dbl} {"Fs"=1000.0, "#s"=1000.0} ("sampling info"), "Fs"=w907, "#s"=w915) -> (w916:cluster{"Fs":dbl, "#s":dbl})
                                n405 = call <vilib>:"Sine Waveform.vi"("offset"=0.0, "sampling info"=w916, "reset signal"=TRUE, "amplitude"=w901, "frequency"=w908) -> ("signal out"=w903:waveform(dbl))  [unwired: 5 in, 1 out]
                                n406 = case shown="真" w904 {
                                tunnel: w903 -> [w917 w919]
                                tunnel: [w917 w918] -> w902
                                frame False {
                                }
                                frame True {
                                n407 = Negate(x=w919) -> (-x=w918:waveform(dbl))
                                }
                                }
                                n408 = Add(x=w902, y=w901) -> (x+y=w900:waveform(dbl))
                                }
                                frame #1 {
                                n409 = Divide(x=w929, y=w930) -> (x/y=w935:dbl)
                                n410 = Multiply(x=w935, y=w920) -> (x*y=w936:dbl)
                                n411 = Divide(x=w921, y=2.0) -> (x/y=w925:dbl)
                                n412 = local read "完\n整\n缺\n齿\n波"() -> (w922:waveform(dbl))
                                n413 = Bundle By Name(cluster=cluster{"Fs":dbl, "#s":dbl} {"Fs"=1000.0, "#s"=1000.0} ("sampling info"), "Fs"=w929, "#s"=w936) -> (w937:cluster{"Fs":dbl, "#s":dbl})
                                n414 = call <vilib>:"Sine Waveform.vi"("offset"=0.0, "sampling info"=w937, "reset signal"=TRUE, "amplitude"=w925, "frequency"=w930) -> ("signal out"=w927:waveform(dbl))  [unwired: 5 in, 1 out]
                                n415 = case shown="真" w928 {
                                tunnel: w927 -> [w941 w945]
                                tunnel: [w938 w945] -> w926
                                tunnel: [w943 w946] -> w923
                                tunnel: w922 -> [w944 w946]
                                tunnel: w921 -> [w940 _]
                                frame False {
                                n416 = Negate(x=w941) -> (-x=w939:waveform(dbl))
                                n417 = Negate(x=w944) -> (-x=w942:waveform(dbl))
                                n418 = Add(x=w939, y=w940) -> (x+y=w938:waveform(dbl))
                                n419 = Add(x=w940, y=w942) -> (x+y=w943:waveform(dbl))
                                }
                                frame True {
                                }
                                }
                                n420 = Add(x=w926, y=w925) -> (x+y=w924:waveform(dbl))
                                }
                              }
                              n421 = call "拼接信号23"("Input Signal B"=w896, "Input Signal A"=w890) -> ("Appended Signals"=w894:dynamicdata)  [unwired: 8 in, 1 out]
                              n422 = call "拼接信号24"("Input Signal B"=w894, "Input Signal A"=w889) -> ("Appended Signals"=w892:dynamicdata)  [unwired: 8 in, 1 out]
                            }
                          }
                        }
                      }
                      n423 = case shown="真" w846 {
                        tunnel: w845 -> [_ w870]
                        tunnel: [_ w869] -> w844
                        tunnel: w842 -> [_ w868]
                        frame False {
                        }
                        frame True {
                          n424 = stacked-sequence {
                            tunnel: w870 -> [w871 w873 _]
                            tunnel: [_ _ w877] -> w869
                            tunnel: w868 -> [_ w872 _]
                            frame #0 {
                              n425 = local write "曲轴圈数信号"(w871) -> ()
                            }
                            frame #1 {
                              n426 = for {
                                N: w872 -> [_]
                                tunnel: w873 -> [w876]
                                n427 = local read "曲轴圈数信号"() -> (w875:dynamicdata)
                                n428 = call "拼接信号18"("Input Signal B"=w876, "Input Signal A"=w875) -> ("Appended Signals"=w874:dynamicdata)  [unwired: 8 in, 1 out]
                                n429 = local write "曲轴圈数信号"(w874) -> ()
                              }
                            }
                            frame #2 {
                              n430 = local read "曲轴圈数信号"() -> (w877:dynamicdata)
                            }
                          }
                        }
                      }
                      n431 = Bundle By Name("Y"=dbl[] []) -> (w862:waveform(dbl))  [unwired: 1 in]
                      n432 = case shown="4" w852 {
                        tunnel: w844 -> [w948 w952 w959]
                        tunnel: [w948 w952 w956] -> w865
                        tunnel: w856 -> [_ w950 w961]
                        tunnel: [w947 w951 w960] -> w863
                        tunnel: w862 -> [w947 w949 w957]
                        tunnel: [w947 w949 w958] -> w861
                        tunnel: [w947 w949 w959] -> w860
                        tunnel: [w947 w949 w957] -> w859
                        tunnel: w850 -> [_ _ _]
                        tunnel: w854 -> [_ _ w956]
                        frame 1 {
                        }
                        frame 2, Default {
                          n433 = Negate(x=w952) -> (-x=w953:dynamicdata)
                          n434 = Add(x=w953, y=w950) -> (x+y=w951:dynamicdata)
                        }
                        frame 4 {
                          n435 = Negate(x=w956) -> (-x=w955:dynamicdata)
                          n436 = Negate(x=w959) -> (-x=w954:dynamicdata)
                          n437 = Add(x=w961, y=w954) -> (x+y=w958:dynamicdata)
                          n438 = Add(x=w955, y=w961) -> (x+y=w960:dynamicdata)
                        }
                      }
                      "5波形图" <- w861
                      "6波形图" <- w860
                    }
                  }
                }
                frame 1 {
                  n439 = stacked-sequence {
                    tunnel: w975 -> [w987 w1003 w1030]
                    tunnel: w974 -> [w986 w1017 _]
                    tunnel: w973 -> [w980 w1016 _]
                    tunnel: w972 -> [w985 _ _]
                    tunnel: w971 -> [_ _ w1038]
                    tunnel: [_ _ w1035] -> w970
                    tunnel: [_ _ w1036] -> w969
                    tunnel: w968 -> [_ _ w1040]
                    tunnel: w967 -> [w978 _ _]
                    tunnel: w966 -> [_ w1012 _]
                    tunnel: [w977 _ _] -> w963
                    tunnel: [_ _ w1036] -> w965
                    tunnel: w964 -> [_ _ w1031]
                    tunnel: [_ _ w1029] -> w962
                    frame #0 {
                      n440 = Equal To 0?(x=w980) -> (x = 0?=w979:bool)
                      n441 = Divide(x=w986, y=w980) -> (x/y=w992:dbl)
                      n442 = Multiply(x=w992, y=w985) -> (x*y=w993:dbl)
                      n443 = case shown="假" w979 {
                        tunnel: w980 -> [w1001 _]
                        tunnel: w978 -> [w999 _]
                        tunnel: [w995 0.0] -> w976
                        frame False {
                          n444 = Reciprocal(x=w1001) -> (1/x=w1000:dbl)
                          n445 = Multiply(x=w999, y=w1000) -> (x*y=w998:dbl)
                          n446 = Reciprocal(x=w998) -> (1/x=w997:dbl)
                          n447 = Multiply(x=w997, y=60.0) -> (x*y=w995:dbl)
                        }
                        frame True {
                        }
                      }
                      n448 = Divide(x=w987, y=2.0) -> (x/y=w982:dbl)
                      "曲轴方波偏移量" <- w982
                      n449 = Bundle By Name(cluster=cluster{"Fs":dbl, "#s":dbl} {"Fs"=1000.0, "#s"=1000.0} ("sampling info"), "Fs"=w986, "#s"=w993) -> (w994:cluster{"Fs":dbl, "#s":dbl})
                      n450 = call <vilib>:"Square Waveform.vi"("duty cycle (%)"=50.0, "offset"=0.0, "sampling info"=w994, "reset signal"=TRUE, "amplitude"=w982, "frequency"=w980) -> ("signal out"=w983:waveform(dbl))  [unwired: 4 in, 1 out]
                      n451 = Add(x=w982, y=w983) -> (x+y=→"曲轴方波波形图":waveform(dbl))
                      n452 = Round To Nearest(number=w976) -> (nearest integer value=w977:dbl)
                    }
                    frame #1 {
                      n453 = Divide(x=w1017, y=w1016) -> (x/y=w1014:dbl)
                      n454 = Divide(x=w1017, y=w1016) -> (x/y=w1026:dbl)
                      n455 = Multiply(x=w1014, y=w1012) -> (x*y=w1013:dbl)
                      n456 = Multiply(x=w1026, y=0.5) -> (x*y=w1027:dbl)
                      n457 = Bundle By Name(cluster=cluster{"Fs":dbl, "#s":dbl} {"Fs"=1000.0, "#s"=1000.0} ("sampling info"), "Fs"=w1017, "#s"=w1027) -> (w1028:cluster{"Fs":dbl, "#s":dbl})
                      n458 = Bundle By Name(cluster=cluster{"Fs":dbl, "#s":dbl} {"Fs"=1000.0, "#s"=1000.0} ("sampling info"), "Fs"=w1017, "#s"=w1013) -> (w1021:cluster{"Fs":dbl, "#s":dbl})
                      n459 = Divide(x=w1003, y=2.0) -> (x/y=w1005:dbl)
                      n460 = call <vilib>:"Square Waveform.vi"("duty cycle (%)"=50.0, "offset"=w1005, "sampling info"=w1028, "reset signal"=TRUE, "amplitude"=w1005, "frequency"=w1016) -> ("signal out"=w1008:waveform(dbl))  [unwired: 4 in, 1 out]
                      n461 = call <vilib>:"Square Waveform.vi"("duty cycle (%)"=100.0, "offset"=w1003, "sampling info"=w1021, "reset signal"=TRUE, "amplitude"=0.0, "frequency"=w1016) -> ("signal out"=w1007:waveform(dbl))  [unwired: 4 in, 1 out]
                      n462 = Negate(x=w1008) -> (-x=w1006:waveform(dbl))
                      n463 = call "拼接信号15"("Input Signal B"=w1007, "Input Signal A"=w1008) -> ("Appended Signals"=w1011:dynamicdata)  [unwired: 8 in, 1 out]
                      n464 = Add(x=w1003, y=w1006) -> (x+y=w1004:waveform(dbl))
                      n465 = call "拼接信号39"("Input Signal B"=w1004, "Input Signal A"=w1011) -> ("Appended Signals"=→"曲轴方波缺齿波形图":dynamicdata)  [unwired: 8 in, 1 out]
                    }
                    frame #2 {
                      n466 = local read "曲轴方波缺齿波形图"() -> (w1042:dynamicdata)
                      n467 = local read "曲轴方波波形图"() -> (w1043:waveform(dbl))
                      n468 = Greater Than 0?(x=w1031) -> (x > 0?=w1032:bool)
                      n469 = call "拼接信号16"("Input Signal B"=w1042, "Input Signal A"=w1043) -> ("Appended Signals"=w1029:dynamicdata)  [unwired: 8 in, 1 out]
                      n470 = Decrement(x=w1031) -> (x-1=w1034:dbl)
                      n471 = case shown="真" w1032 {
                        tunnel: w1029 -> [_ w1046]
                        tunnel: w1034 -> [_ w1045]
                        tunnel: [_ w1044] -> w1033
                        frame False {
                        }
                        frame True {
                          n472 = stacked-sequence {
                            tunnel: w1046 -> [w1047 w1049 _]
                            tunnel: w1045 -> [_ w1048 _]
                            tunnel: [_ _ w1053] -> w1044
                            frame #0 {
                              n473 = local write "曲轴组合波形"(w1047) -> ()
                            }
                            frame #1 {
                              n474 = for {
                                N: w1048 -> [_]
                                tunnel: w1049 -> [w1051]
                                n475 = local read "曲轴组合波形"() -> (w1052:waveform(dbl))
                                n476 = call "拼接信号17"("Input Signal B"=w1051, "Input Signal A"=w1052) -> ("Appended Signals"=w1050:dynamicdata)  [unwired: 8 in, 1 out]
                                n477 = local write "曲轴组合波形"(w1050) -> ()
                              }
                            }
                            frame #2 {
                              n478 = local read "曲轴组合波形"() -> (w1053:waveform(dbl))
                            }
                          }
                        }
                      }
                      n479 = case shown="真" w1038 {
                        tunnel: w1033 -> [w1054 w1058]
                        tunnel: [w1054 w1056] -> w1037
                        tunnel: w1030 -> [_ w1055]
                        frame False {
                        }
                        frame True {
                          n480 = Negate(x=w1058) -> (-x=w1057:waveform(dbl))
                          n481 = Add(x=w1057, y=w1055) -> (x+y=w1056:waveform(dbl))
                        }
                      }
                      n482 = Bundle By Name("Y"=dbl[] []) -> (w1036:waveform(dbl))  [unwired: 1 in]
                      n483 = case shown="2" w1040 {
                        tunnel: w1037 -> [w1060 w1061]
                        tunnel: [w1060 w1062] -> w1035
                        tunnel: w1030 -> [_ w1063]
                        tunnel: [w1059 w1061] -> w1039
                        tunnel: w1036 -> [w1059 _]
                        frame 1, Default {
                        }
                        frame 2 {
                          n484 = Negate(x=w1061) -> (-x=w1064:waveform(dbl))
                          n485 = Add(x=w1064, y=w1063) -> (x+y=w1062:waveform(dbl))
                        }
                      }
                      "1波形图" <- w1039
                    }
                  }
                }
                frame 2 {
                  n486 = Bundle By Name("Y"=dbl[] []) -> (w1066:waveform(dbl))  [unwired: 1 in]
                }
              }
              "Hall Channel 2" <- w8
              "ME Channel 1" <- w12
              "ME Channel 2" <- w21
              "转速表" <- w25
              n487 = call "从动态数据转换5"("Dynamic Data Type"=w7) -> ()  [unwired: 3 in, 1 out]
              n488 = property on="AO2 Channel" class="Ring (严格)"() -> ("Value"=w15:u32)  [unwired: 2 in, 2 out]
              n489 = property on="AO0 Channel" class="Ring (严格)"() -> ("Value"=w24:u32)  [unwired: 2 in, 2 out]
              n490 = property on="AO1 Channel" class="Ring (严格)"() -> ("Value"=w23:u32)  [unwired: 2 in, 2 out]
              n491 = property on="AO3 Channel" class="Ring (严格)"() -> ("Value"=w14:u32)  [unwired: 2 in, 2 out]
              n492 = case shown="5" w14 {
                tunnel: w4 -> [w74 _ _ _ _ _]
                tunnel: [w74 w75 w76 w77 w78 w79] -> w18
                tunnel: w8 -> [_ w75 _ _ _ _]
                tunnel: w21 -> [_ _ _ w77 _ _]
                tunnel: w6 -> [_ _ _ _ w78 _]
                tunnel: w20 -> [_ _ _ _ _ w79]
                tunnel: w12 -> [_ _ w76 _ _ _]
                frame 0 {
                }
                frame 1 {
                }
                frame 2, Default {
                }
                frame 3 {
                }
                frame 4 {
                }
                frame 5 {
                }
              }
              n493 = case shown="5" w15 {
                tunnel: w4 -> [w80 _ _ _ _ _]
                tunnel: [w80 w81 w82 w83 w84 w85] -> w19
                tunnel: w8 -> [_ w81 _ _ _ _]
                tunnel: w21 -> [_ _ _ w83 _ _]
                tunnel: w6 -> [_ _ _ _ w84 _]
                tunnel: w20 -> [_ _ _ _ _ w85]
                tunnel: w12 -> [_ _ w82 _ _ _]
                frame 0 {
                }
                frame 1 {
                }
                frame 2, Default {
                }
                frame 3 {
                }
                frame 4 {
                }
                frame 5 {
                }
              }
              n494 = case shown="2, 默认" w23 {
                tunnel: w4 -> [w86 _ _ _ _ _]
                tunnel: [w86 w87 w88 w89 w90 w91] -> w28
                tunnel: w12 -> [_ _ w88 _ _ _]
                tunnel: w21 -> [_ _ _ w89 _ _]
                tunnel: w6 -> [_ _ _ _ w90 _]
                tunnel: w20 -> [_ _ _ _ _ w91]
                tunnel: w8 -> [_ w87 _ _ _ _]
                frame 0 {
                }
                frame 1 {
                }
                frame 2, Default {
                }
                frame 3 {
                }
                frame 4 {
                }
                frame 5 {
                }
              }
              n495 = case shown="0" w24 {
                tunnel: w4 -> [w92 _ _ _ _ _]
                tunnel: [w92 w93 w94 w95 w96 w97] -> w29
                tunnel: w8 -> [_ w93 _ _ _ _]
                tunnel: w12 -> [_ _ w94 _ _ _]
                tunnel: w21 -> [_ _ _ w95 _ _]
                tunnel: w6 -> [_ _ _ _ w96 _]
                tunnel: w20 -> [_ _ _ _ _ w97]
                frame 0 {
                }
                frame 1 {
                }
                frame 2, Default {
                }
                frame 3 {
                }
                frame 4 {
                }
                frame 5 {
                }
              }
              n496 = call "从动态数据转换9"("Dynamic Data Type"=w29) -> ("Array"=w27:dbl[])  [unwired: 3 in]
              n497 = call "从动态数据转换10"("Dynamic Data Type"=w28) -> ("Array"=w26:dbl[])  [unwired: 3 in]
              n498 = call "从动态数据转换3"("Dynamic Data Type"=w19) -> ("Array"=w17:dbl[])  [unwired: 3 in]
              n499 = call "从动态数据转换4"("Dynamic Data Type"=w18) -> ("Array"=w16:dbl[])  [unwired: 3 in]
              n500 = Build Array(w27, w26, w17, w16) -> ()  [unwired: 1 out]
            }
          }
          frame "停止" {
            n501 = One Button Dialog(message="程序已停止" ("消息")) -> ()  [unwired: 1 in, 1 out]
          }
          frame "编辑" {
            n502 = call-by-ref "?"() -> ("品牌"=w1089:string, "车型"=w1088:string, "曲轴信号类型"=w1070:dbl, "曲轴个数"=w1085:dbl, "曲轴圈数"=w1087:dbl, "曲轴电压幅值"=w1084:dbl, "总齿数"=w1086:dbl, "缺齿数"=w1083:dbl, "缺齿偏移"=w1072:dbl, "曲轴是否取反"=w1071:dbl, "凸轮轴信号类型"=w1074:dbl, "凸轮轴个数"=w1082:dbl, "信号个数"=w1075:dbl, "凸轮轴周期"=w1081:dbl, "凸轮轴电压幅值"=w1080:dbl, "起始偏移"=w1079:dbl, "间隔齿数"=w1078:dbl, "插齿间隔"=w1077:dbl, "凸轮轴是否取反"=w1076:dbl, "OK"=w1073:bool)  [unwired: 9 in, 3 out]
            n503 = Not Equal?(x=w1089, y="") -> (x != y?=w1094:bool)
            n504 = And(x=w1073, y=w1094) -> (x .and. y?=w1091:bool)
            n505 = Not Equal?(x=w1088, y="") -> (x != y?=w1092:bool)
            n506 = And(x=w1091, y=w1092) -> (x .and. y?=w1090:bool)
            "数值合法" <- w1090
            n507 = case shown="真" w1090 {
              tunnel: w1089 -> [w1098 w1127]
              tunnel: w1088 -> [w1097 w1126]
              tunnel: w1085 -> [_ w1125]
              tunnel: w1070 -> [_ w1124]
              tunnel: w1087 -> [_ w1123]
              tunnel: w1086 -> [_ w1122]
              tunnel: w1072 -> [_ w1121]
              tunnel: w1084 -> [_ w1120]
              tunnel: w1083 -> [_ w1119]
              tunnel: w1071 -> [_ w1118]
              tunnel: w1082 -> [_ w1117]
              tunnel: w1081 -> [_ w1116]
              tunnel: w1080 -> [_ w1115]
              tunnel: w1079 -> [_ w1114]
              tunnel: w1078 -> [_ w1113]
              tunnel: w1077 -> [_ w1112]
              tunnel: w1076 -> [_ w1111]
              tunnel: w1075 -> [_ w1110]
              tunnel: w1074 -> [_ w1109]
              tunnel: w1073 -> [w1096 _]
              frame False {
                n508 = Equal?(x=w1098, y="") -> (x = y?=w1100:bool)
                n509 = Equal?(x=w1097, y="") -> (x = y?=w1101:bool)
                n510 = And(x=w1096, y=w1100) -> (x .and. y?=w1099:bool)
                n511 = case shown="假" w1099 {
                  tunnel: w1101 -> [w1106 _]
                  tunnel: w1096 -> [w1104 _]
                  frame False {
                    n512 = And(x=w1104, y=w1106) -> (x .and. y?=w1105:bool)
                    n513 = case shown="真" w1105 {
                      frame False {
                      }
                      frame True {
                        n514 = One Button Dialog(message="车型不能为空" ("消息")) -> ()  [unwired: 1 in, 1 out]
                      }
                    }
                  }
                  frame True {
                    n515 = One Button Dialog(message="品牌不能为空" ("消息")) -> ()  [unwired: 1 in, 1 out]
                  }
                }
              }
              frame True {
                n516 = stacked-sequence {
                  tunnel: w1127 -> [w1130 _ _]
                  tunnel: w1126 -> [w1129 _ _]
                  tunnel: w1125 -> [_ w1138 _]
                  tunnel: w1124 -> [_ w1137 _]
                  tunnel: w1123 -> [_ w1136 _]
                  tunnel: w1122 -> [_ w1132 _]
                  tunnel: w1121 -> [_ w1135 _]
                  tunnel: w1120 -> [_ w1134 _]
                  tunnel: w1119 -> [_ w1133 _]
                  tunnel: w1118 -> [_ w1131 _]
                  tunnel: w1117 -> [_ _ w1167]
                  tunnel: w1116 -> [_ _ w1166]
                  tunnel: w1115 -> [_ _ w1165]
                  tunnel: w1114 -> [_ _ w1164]
                  tunnel: w1113 -> [_ _ w1163]
                  tunnel: w1112 -> [_ _ w1162]
                  tunnel: w1111 -> [_ _ w1161]
                  tunnel: w1110 -> [_ _ w1160]
                  tunnel: w1109 -> [_ _ w1159]
                  frame #0 {
                    n517 = Build Array(w1130, w1129) -> (→"品牌车型数组":string[])
                  }
                  frame #1 {
                    n518 = stacked-sequence {
                      tunnel: w1131 -> [w1147 _]
                      tunnel: w1136 -> [w1145 _]
                      tunnel: w1134 -> [w1144 _]
                      tunnel: w1132 -> [w1143 _]
                      tunnel: w1133 -> [w1142 _]
                      tunnel: w1135 -> [w1141 _]
                      tunnel: w1138 -> [w1140 _]
                      tunnel: w1137 -> [w1139 _]
                      frame #0 {
                        n519 = case shown="1" w1147 {
                          tunnel: [FALSE TRUE] -> w1146
                          frame 0, Default {
                          }
                          frame 1 {
                          }
                        }
                        "0曲轴是否取反" <- w1146
                        "0曲轴轴信号类型" <- w1139
                        "0曲轴电压幅值" <- w1144
                        "0总齿数" <- w1143
                        "0曲轴个数" <- w1140
                        "0缺齿数" <- w1142
                        "0曲轴圈数" <- w1145
                        "0缺齿偏移" <- w1141
                      }
                      frame #1 {
                        n520 = local read "0曲轴轴信号类型"() -> (w1151:u32)
                        n521 = local read "0曲轴圈数"() -> (w1157:dbl)
                        n522 = local read "0缺齿偏移"() -> (w1158:dbl)
                        n523 = local read "0曲轴电压幅值"() -> (w1152:dbl)
                        n524 = local read "0总齿数"() -> (w1153:dbl)
                        n525 = local read "0曲轴个数"() -> (w1154:dbl)
                        n526 = local read "0曲轴是否取反"() -> (w1155:bool)
                        n527 = local read "0缺齿数"() -> (w1156:dbl)
                        n528 = Bundle("0曲轴轴信号类型"=w1151, "0曲轴电压幅值"=w1152, "0总齿数"=w1153, "0曲轴个数"=w1154, "0曲轴是否取反"=w1155, "0缺齿数"=w1156, "0曲轴圈数"=w1157, "0缺齿偏移"=w1158) -> (→"曲轴参数":T4)  [unwired: 1 in]
                      }
                    }
                  }
                  frame #2 {
                    n529 = stacked-sequence {
                      tunnel: w1166 -> [w1177 _]
                      tunnel: w1165 -> [w1176 _]
                      tunnel: w1164 -> [w1175 _]
                      tunnel: w1163 -> [w1174 _]
                      tunnel: w1162 -> [w1173 _]
                      tunnel: w1161 -> [w1172 _]
                      tunnel: w1160 -> [w1170 _]
                      tunnel: w1159 -> [w1169 _]
                      tunnel: w1167 -> [w1168 _]
                      frame #0 {
                        n530 = case shown="0, 默认" w1172 {
                          tunnel: [FALSE TRUE] -> w1171
                          frame 0, Default {
                          }
                          frame 1 {
                          }
                        }
                        "0凸轮轴是否取反" <- w1171
                        "0凸轮轴信号类型" <- w1169
                        "0凸轮轴电压幅值" <- w1176
                        "0信号个数" <- w1170
                        "0凸轮轴个数" <- w1168
                        "0凸轮轴周期" <- w1177
                        "0起始偏移" <- w1175
                        "0插齿间隔" <- w1173
                        "0间隔齿数" <- w1174
                      }
                      frame #1 {
                        n531 = local read "0凸轮轴信号类型"() -> (w1181:u32)
                        n532 = local read "0凸轮轴电压幅值"() -> (w1182:dbl)
                        n533 = local read "0信号个数"() -> (w1183:dbl)
                        n534 = local read "0凸轮轴个数"() -> (w1184:dbl)
                        n535 = local read "0凸轮轴是否取反"() -> (w1185:bool)
                        n536 = local read "0凸轮轴周期"() -> (w1186:dbl)
                        n537 = local read "0起始偏移"() -> (w1187:dbl)
                        n538 = local read "0插齿间隔"() -> (w1188:dbl)
                        n539 = local read "0间隔齿数"() -> (w1189:dbl)
                        n540 = Bundle("0凸轮轴信号类型"=w1181, "0凸轮轴电压幅值"=w1182, "0信号个数"=w1183, "0凸轮轴个数"=w1184, "0凸轮轴是否取反"=w1185, "0凸轮轴周期"=w1186, "0起始偏移"=w1187, "0插齿间隔"=w1188, "0间隔齿数"=w1189) -> (→"凸轮轴参数":T1)  [unwired: 1 in]
                      }
                    }
                  }
                }
              }
            }
          }
          frame "保存" {
            n541 = local read "数值合法"() -> (w1194:bool)
            n542 = Equal?(x=w1190, y="保存") -> (x = y?=w1191:bool)
            n543 = And(x=w1191, y=w1194) -> (x .and. y?=w1193:bool)
            n544 = case shown="真" w1193 {
              frame False {
                n545 = One Button Dialog(message="未编辑信号参数" ("消息")) -> ()  [unwired: 1 in, 1 out]
              }
              frame True {
                n546 = stacked-sequence {
                  frame #0 {
                    n547 = stacked-sequence {
                      frame #0 {
                        n548 = local read "品牌车型数组"() -> (w1199:string[])
                        n549 = Index Array(array=w1199, index=0 ("索引")) -> (element=w1202:string)
                        "品牌" <- w1202
                        n550 = Index Array(array=w1199, index=1 ("索引")) -> (element=w1198:string)
                        n551 = Current VI's Path() -> (path=w1209:path)
                        n552 = Strip Path(path=w1209) -> (stripped path=w1208:path)  [unwired: 1 out]
                        n553 = Build Path(base path=w1208, name or relative path="品牌文件" ("名称或相对路径")) -> (appended path=w1204:path)
                        n554 = Concatenate Strings(w1202, ".xml") -> (w1205:string)
                        n555 = Build Array(w1198) -> (w1197:string[])
                        "车型数组" <- w1197
                        n556 = Build Path(base path=w1204, name or relative path=w1205) -> (appended path=w1203:path)
                        n557 = Flatten To XML(6:w1197) -> (2:w1196:string)
                        n558 = call-poly <vilib>:"Write to XML File.vi"("Standalone? (T)"=TRUE, "XML Encoding"="GB2312", "XML Input"=w1196, "XML File Path"=w1203) -> ()  [unwired: 5 in, 3 out]
                      }
                      frame #1 {
                        n559 = stacked-sequence {
                          frame #0 {
                            n560 = Current VI's Path() -> (path=w1223:path)
                            n561 = Strip Path(path=w1223) -> (stripped path=w1222:path)  [unwired: 1 out]
                            n562 = Build Path(base path=w1222, name or relative path="品牌文件" ("名称或相对路径")) -> (appended path=w1217:path)
                            n563 = Concatenate Strings("品牌" ("字符串"), ".xml") -> (w1216:string)
                            n564 = Build Path(base path=w1217, name or relative path=w1216) -> (appended path=w1215:path)
                            n565 = call-poly <vilib>:"Read From XML File.vi"("error in (no error)"="error", "XML File Path"=w1215) -> ("error out"=w1225:errorcluster, "XML Elements"=w1224:string)  [unwired: 7 in, 1 out]
                            n566 = Unflatten From XML(xml string=w1224, type="字符串数组类型", error in (no error)=w1225) -> (value=w1213:string[])  [unwired: 1 out]
                            "品牌数组" <- w1213
                            n567 = Array Size(array=w1213) -> (size(s)=→"数组大小":i32)
                          }
                          frame #1 {
                            n568 = local read "品牌数组"() -> (w1228:string[])
                            n569 = local read "品牌"() -> (w1229:string)
                            n570 = local read "数组大小"() -> (w1227:i32)
                            n571 = Insert Into Array(array=w1228, index=w1227, new element=w1229) -> (w1226:string[])
                            n572 = local write "品牌数组"(w1226) -> ()
                          }
                          frame #2 {
                            n573 = Current VI's Path() -> (path=w1240:path)
                            n574 = Strip Path(path=w1240) -> (stripped path=w1239:path)  [unwired: 1 out]
                            n575 = Build Path(base path=w1239, name or relative path="品牌文件" ("名称或相对路径")) -> (appended path=w1235:path)
                            n576 = Concatenate Strings("品牌", ".xml") -> (w1236:string)
                            n577 = local read "品牌数组"() -> (w1231:string[])
                            n578 = Build Path(base path=w1235, name or relative path=w1236) -> (appended path=w1234:path)
                            n579 = Flatten To XML(6:w1231) -> (2:w1230:string)
                            n580 = call-poly <vilib>:"Write to XML File.vi"("Standalone? (T)"=TRUE, "XML Encoding"="GB2312", "XML Input"=w1230, "XML File Path"=w1234) -> ()  [unwired: 5 in, 3 out]
                          }
                        }
                      }
                    }
                  }
                  frame #1 {
                    w1255 = "Camshaft_Signal" ("section")
                    w1301 = "Crank_Signal" ("section")
                    n581 = local read "曲轴参数"() -> (w1332:T2)
                    n582 = local read "凸轮轴参数"() -> (w1283:T1)
                    n583 = Current VI's Path() -> (path=w1298:path)
                    n584 = Unbundle(w1332) -> ("0曲轴轴信号类型"=w1329:u32, "0曲轴电压幅值"=w1327:dbl, "0总齿数"=w1326:dbl, "0曲轴个数"=w1325:dbl, "0曲轴是否取反"=w1328:bool, "0却齿数"=w1330:dbl, "0曲轴圈数"=w1331:dbl, "0缺齿偏移"=w1242:dbl)
                    n585 = Strip Path(path=w1298) -> (stripped path=w1297:path)  [unwired: 1 out]
                    n586 = Unbundle(w1283) -> ("0凸轮轴信号类型"=w1275:u32, "0凸轮轴电压幅值"=w1281:dbl, "0信号个数"=w1276:dbl, "0凸轮轴个数"=w1274:dbl, "0凸轮轴是否取反"=w1277:bool, "0凸轮轴周期"=w1282:dbl, "0起始偏移"=w1280:dbl, "0插齿间隔"=w1278:dbl, "0间隔齿数"=w1279:dbl)
                    n587 = local read "品牌车型数组"() -> (w1288:string[])
                    n588 = Index Array(array=w1288, index=1 ("索引")) -> (element=w1289:string)
                    n589 = Index Array(array=w1288, index=0 ("索引")) -> (element=w1291:string)
                    n590 = Build Path(base path=w1297, name or relative path="曲轴凸轮轴配置文件" ("名称或相对路径")) -> (appended path=w1295:path)
                    n591 = Concatenate Strings(w1289, ".ini" ("字符串")) -> (w1293:string)
                    n592 = Build Path(base path=w1295, name or relative path=w1291) -> (appended path=w1286:path)
                    n593 = String To Path(string=w1293) -> (path=w1287:path)
                    n594 = Create Folder(path (use dialog)=w1286) -> (created path=w1284:path)  [unwired: 2 in, 2 out]
                    n595 = Build Path(base path=w1284, name or relative path=w1287) -> (appended path=w1285:path)
                    n596 = call <vilib>:"Open Config Data.vi"("create file if necessary (T)"=TRUE ("create file if necessary? (T)"), "configuration file path"=w1285) -> ("error out"=w1321:errorcluster, "refnum"=w1319:T3)  [unwired: 7 in, 1 out]
                    n597 = call-poly <vilib>:"Write Key.vi"("section"=w1301, "error in (no error)"=w1321, "value"=w1329, "key"="type", "refnum"=w1319) -> ("error out"=w1322:errorcluster, "refnum out"=w1320:T3)  [unwired: 4 in, 1 out]
                    n598 = call-poly <vilib>:"Write Key.vi"("section"=w1301, "error in (no error)"=w1322, "value"=w1327, "key"="voltage" ("键2"), "refnum"=w1320) -> ("error out"=w1317:errorcluster, "refnum out"=w1316:T3)  [unwired: 4 in, 1 out]
                    n599 = call-poly <vilib>:"Write Key.vi"("section"=w1301, "error in (no error)"=w1317, "value"=w1328, "key"="invert" ("键3"), "refnum"=w1316) -> ("error out"=w1314:errorcluster, "refnum out"=w1313:T3)  [unwired: 4 in, 1 out]
                    n600 = call-poly <vilib>:"Write Key.vi"("section"=w1301, "error in (no error)"=w1314, "value"=w1325, "key"="crank_number" ("键3"), "refnum"=w1313) -> ("error out"=w1311:errorcluster, "refnum out"=w1310:T3)  [unwired: 4 in, 1 out]
                    n601 = call-poly <vilib>:"Write Key.vi"("section"=w1301, "error in (no error)"=w1311, "value"=w1326, "key"="tooth_number" ("键3"), "refnum"=w1310) -> ("error out"=w1308:errorcluster, "refnum out"=w1309:T3)  [unwired: 4 in, 1 out]
                    n602 = call-poly <vilib>:"Write Key.vi"("section"=w1301, "error in (no error)"=w1308, "value"=w1330, "key"="edentulous_number" ("键3"), "refnum"=w1309) -> ("error out"=w1305:errorcluster, "refnum out"=w1304:T3)  [unwired: 4 in, 1 out]
                    n603 = call-poly <vilib>:"Write Key.vi"("section"=w1301, "error in (no error)"=w1305, "value"=w1331, "key"="cylinder_number" ("键3"), "refnum"=w1304) -> ("error out"=w1300:errorcluster, "refnum out"=w1302:T3)  [unwired: 4 in, 1 out]
                    n604 = call-poly <vilib>:"Write Key.vi"("section"=w1301, "error in (no error)"=w1300, "value"=w1242, "key"="edentulous_offset" ("键2"), "refnum"=w1302) -> ("error out"=w1244:errorcluster, "refnum out"=w1245:T3)  [unwired: 4 in, 1 out]
                    n605 = call-poly <vilib>:"Write Key.vi"("section"=w1255, "error in (no error)"=w1244, "value"=w1275, "key"="type" ("键3"), "refnum"=w1245) -> ("error out"=w1273:errorcluster, "refnum out"=w1272:T3)  [unwired: 4 in, 1 out]
                    n606 = call-poly <vilib>:"Write Key.vi"("section"=w1255, "error in (no error)"=w1273, "value"=w1281, "key"="voltage" ("键3"), "refnum"=w1272) -> ("error out"=w1270:errorcluster, "refnum out"=w1268:T3)  [unwired: 4 in, 1 out]
                    n607 = call-poly <vilib>:"Write Key.vi"("section"=w1255, "error in (no error)"=w1270, "value"=w1276, "key"="signal_number" ("键3"), "refnum"=w1268) -> ("error out"=w1264:errorcluster, "refnum out"=w1267:T3)  [unwired: 4 in, 1 out]
                    n608 = call-poly <vilib>:"Write Key.vi"("section"=w1255, "error in (no error)"=w1264, "value"=w1274, "key"="camshaft_number" ("键3"), "refnum"=w1267) -> ("error out"=w1269:errorcluster, "refnum out"=w1266:T3)  [unwired: 4 in, 1 out]
                    n609 = call-poly <vilib>:"Write Key.vi"("section"=w1255, "error in (no error)"=w1269, "value"=w1277, "key"="invert" ("键2"), "refnum"=w1266) -> ("error out"=w1271:errorcluster, "refnum out"=w1265:T3)  [unwired: 4 in, 1 out]
                    n610 = call-poly <vilib>:"Write Key.vi"("section"=w1255, "error in (no error)"=w1271, "value"=w1282, "key"="cycle", "refnum"=w1265) -> ("error out"=w1260:errorcluster, "refnum out"=w1263:T3)  [unwired: 4 in, 1 out]
                    n611 = call-poly <vilib>:"Write Key.vi"("section"=w1255, "error in (no error)"=w1260, "value"=w1280, "key"="start_offset" ("键2"), "refnum"=w1263) -> ("error out"=w1261:errorcluster, "refnum out"=w1262:T3)  [unwired: 4 in, 1 out]
                    n612 = call-poly <vilib>:"Write Key.vi"("section"=w1255, "error in (no error)"=w1261, "value"=w1278, "key"="interpolated_interval", "refnum"=w1262) -> ("error out"=w1258:errorcluster, "refnum out"=w1259:T3)  [unwired: 4 in, 1 out]
                    n613 = call-poly <vilib>:"Write Key.vi"("section"=w1255, "error in (no error)"=w1258, "value"=w1279, "key"="interval_tooth_number", "refnum"=w1259) -> ("error out"=w1257:errorcluster, "refnum out"=w1256:T3)  [unwired: 4 in, 1 out]
                    n614 = call <vilib>:"Close Config Data.vi"("error in (no error)"=w1257, "write file if changed (T)"=TRUE ("write configuration file? (T)"), "refnum"=w1256) -> ()  [unwired: 9 out]
                  }
                  frame #2 {
                    n615 = property on="曲轴参数" class="Clust (严格)"() -> ("DefVal"=w1333:T2)  [unwired: 2 in, 2 out]
                    n616 = property on="凸轮轴参数" class="Clust (严格)"() -> ("DefVal"=w1334:T1)  [unwired: 2 in, 2 out]
                    n617 = property on="品牌车型数组" class="Arr (严格)"() -> ("DefVal"=w1335:string[])  [unwired: 2 in, 2 out]
                    n618 = local write "曲轴参数"(w1333) -> ()
                    n619 = local write "凸轮轴参数"(w1334) -> ()
                    n620 = local write "品牌车型数组"(w1335) -> ()
                  }
                  frame #3 {
                    n621 = One Button Dialog(message="保存成功！" ("消息")) -> ()  [unwired: 1 in, 1 out]
                  }
                }
              }
            }
          }
        }
      }
    }
  }
